vi "RG TAS v4c.vi"() -> ()   [LabVIEW 2017]
uses:
  Old Customer Code/Solar fuels TAS - DR/Sub VIs/global tas.vi
  <vilib>/Instr/_visa.llb/VISA Configure Serial Port (Instr).vi
  <vilib>/Analysis/NI_AALPro.lvlib
  <vilib>/Analysis/2dsp.llb/Decimate (single shot, DBL).vi
  <vilib>/Utility/file.llb/Write To Spreadsheet File (DBL).vi
  Optical Software Code Simplified/Modules/Monochromator/Oriel/Oriel (old drivers).lvlib
  Old Customer Code/Solar fuels TAS - DR/Sub VIs/Monochromator/global_Test.vi
  <vilib>/DAQmx/read.llb/DAQmx Read (Analog Wfm 1Chan NSamp).vi
  <vilib>/Analysis/NI_AALBase.lvlib
  <vilib>/Analysis/baseanly.llb/Mean (DBL).vi
  Old Customer Code/Solar fuels TAS - DR/Globals.vi
  <vilib>/Waveform/WDTOps.llb/WDT Index Channel DBL.vi
  <vilib>/Utility/file.llb/Write Delimited Spreadsheet (DBL).vi
panel:
  in  "Inspect Traces":bool
  out "DAQ Loop":i32
  out "Scope Error Counter":i32
  out "Scope time axis":dbl[](array[numeric])
  in  "Stop acquisition":bool
  out "Grating":i32
  in  "2b - Spectrum":bool
  in  "2a - Kinetic":bool
  in  "Stop":bool
  out "Btrace Readout Counter":i32=2
  in  "Stop Btrace Measurement":bool
  out "Readout Counter":i32=2
  in  "Stop Measurement":bool
  in  "Calculate Output Method":T1(ring)=enum."Reflectance"
  in  "Parameters":T2(tab)
  in  "Shutter flow control":u16(ring) items=["None"=0, "XON/XOFF"=1, "RTS/CTS"=2, "DTR/DSR"=4]
  in  "Shutter stop bits":u16(ring)=10 items=["1.0"=10, "1.5"=15, "2.0"=20]
  in  "Shutter parity":u16(ring) items=["None", "Odd", "Even", "Mark", "Space"]
  in  "Shutter data bits":u16=8 min=5 max=8 step=1
  in  "Shutter VISA resource name":refnum<visa-resource-name>="COM1"
  in  "Shutter baud rate":u32=9600
  in  "Shutter open string":string="+100 10\n"
  in  "1 - Move Shutter":bool
  in  "3 - Move mono":bool
  out "Current wavelength (Oriel)":dbl format="%#_13g"
  in  "Monochromator Type":bool=TRUE
  out "Start Wavelength":dbl min=0.0 format="%.3f"
  out "End Wavelength":dbl=100.0 min=0.0 format="%.3f"
  out "Interval Wavelength":dbl=10.0 min=0.0 format="%.3f"
  out "Current Wavelength (PTI)":dbl=300.0 min=300.0 max=2000.0 step=1.0
  in  "Is IR":bool caption="Grating"
  in  "Mono VISA name":refnum<visa-resource-name>
  in  "Mono 2 VISA name":refnum<visa-resource-name>
  out "DAQ dt":dbl=5e-06
  in  "DAQ End Time (s)":dbl=1.0
  in  "DAQ rate":i32=1250000
  in  "DAQ Trigger Level (V)":dbl=0.2
  out "DAQ Number of Samples":dbl=10000.0
  in  "DAQ average number of points":dbl=50.0
  out "DAQ final number of points":dbl
  in  "DAQ Input Channel":tag="Dev1/ai0"
  in  "100% Reflectance Standard (V)":dbl=1.0
  in  "DAQ Card":enum16{"USB-6211", "USB-6251"}(ring)=enum."USB-6251"
  in  "DAQ Input Config":i32(ring)=10106 items=["default"=-1, "RSE"=10083, "NRSE"=10078, "Differential"=10106, "Pseudodifferential"=12529]
  in  "Record Length":u32(ring)=10 items=["1000 points"=1, "10k points"=10, "100k points"=100, "1M points"=1000, "5M points"=5000, "10M points"=10000]
  in  "Acquisition Type":u16(ring)=2 items=["Sample", "Peak Detect", "Hi Res", "Envelope", "Average"]
  in  "Scope average\nnumber of points":dbl=1.0
  in  "Averages on scope":i32=1
  in  "Using TDS Scope?":bool
  in  "CH2 Impedance":u16(ring) items=["1M", "75", "50"]
  in  "CH1 Impedance":u16(ring)=2 items=["1M", "75", "50"]
  in  "Scope VISA resource name":refnum<visa-resource-name>="USB0::0x0699::0x0410::C022077::INSTR"
  in  "Scope Timeout (ms)":u32=30000
  in  "Channel TAS (0: Channel 1)":u16(ring) caption="Channel TAS" items=["Channel 1", "Channel 2", "Channel 3", "Channel 4", "Math", "Reference A", "Reference B", "Reference C", "Reference D"]
  in  "Channel TPC (0: Channel 1)":u16(ring)=1 caption="Channel TPC" items=["Channel 1", "Channel 2", "Channel 3", "Channel 4", "Math", "Reference A", "Reference B", "Reference C", "Reference D"]
  in  "Scope Timebase (per div)":dbl=0.0001 format="%^#_3e"
  in  "Trigger Source":u16(ring)=1 items=["Channel 1", "Channel 2", "Channel 3", "Channel 4", "AC Line", "Aux", "Digital Channel 0", "Digital Channel 1", "Digital Channel 2", "Digital Channel 3", "Digital Channel 4", "Digital Channel 5", "Digital Channel 6", "Digital Channel 7", "Digital Channel 8", "Digital Channel 9", "Digital Channel 10", "Digital Channel 11", "Digital Channel 12", "Digital Channel 13", "Digital Channel 14", "Digital Channel 15", "RF"]
  out "Final number of\nscope points":dbl=10000.0
  in  "Vertical Coupling TAS (1: DC)":u16(ring)=1 caption="Vertical Coupling TAS" items=["AC", "DC", "Ground"]
  in  "Probe Attenuation TAS (10.0)":dbl=1.0 caption="Probe Attenuation TAS"
  in  "Bandwidth CHTAS (0: FULL)":i32(ring) caption="Bandwidth CH TAS" items=["FULL", "250 MHz", "150 MHz", "20 MHz"]
  in  "Vertical Offset CH TAS (0.0 divs)":dbl caption="Vertical Offset CH TAS (in V)"
  in  "Vertical Range CH TAS (10.0 V)":dbl=0.5 caption="Vertical Range CH TAS"
  in  "Trigger Level (V)":dbl=0.25
  in  "Vertical Coupling TPC (1: DC)":u16(ring)=1 caption="Vertical Coupling TPC" items=["AC", "DC", "Ground"]
  in  "Probe Attenuation TPC (1.0)":dbl=1.0 caption="Probe Attenuation TPC"
  in  "Vertical Range TPC (10.0 V)":dbl=0.2 caption="Vertical Range TPC"
  in  "Bandwidth CH TPC (0: FULL)":i32(ring) caption="Bandwidth CH TPC" items=["FULL", "250 MHz", "150 MHz", "20 MHz"]
  in  "Vertical Offset CH TPC (0.0 divs)":dbl caption="Vertical Offset CH TPC (in V)"
  in  "TPC Multiplication factor":dbl=1.0
  out "Number of scope readouts":i32
  in  "Scope Channel Read":bool
  in  "LED on (s)":dbl
  in  "LED off (s)":dbl
  in  "PIA Mode":bool
  in  "LEDs (constant irrad.)":bool caption="LEDs"
  in  "DAQ LED line":string="Dev1/port1/line0"
  in  "Control LEDs?":bool
  out "Scope pretrigger points":dbl=1000.0
  out "Scope CH1 DOD data (A-B final)":waveform(dbl)(graph)
  out "Scope CH1 DOD data (A final)":waveform(dbl)(graph)={"t0"=timestamp(-4.0000000000040004e-05 s since 1904-01-01), "dt"=4.0000000000000003e-07, "Y"=array[10000 elements]}
  out "Scope CH2 data (final)":waveform(dbl)(graph)={"t0"=timestamp(-4.0000000000040004e-05 s since 1904-01-01), "dt"=4.0000000000000003e-07, "Y"=array[10000 elements]}
  out "DAQ DOD data (final)":waveform(dbl)(graph)={"t0"=timestamp(0 s since 1904-01-01), "dt"=5e-06, "Y"=array[10000 elements]}
  out "B trace (Channel1)":waveform(dbl)(graph)
  in  "Amplification Factor":dbl=400.0
  out "Background level (on Amp)":dbl=30.577247161746392
  out "Background level (V)":dbl=0.08993307988748939
  in  "Trace B ?":bool=TRUE
  out "Folder Created":bool
  in  "Sample Name":string="Sample"
  in  "TAS2014  Path":path=path "D:/Solar Fuels Data" caption="Folder"
  out "Path to Files":path=path "D:/Solar Fuels Data/Sample"
  out "Scope Average Channel2":waveform(dbl)(graph)={"t0"=timestamp(-4.0000000000040004e-05 s since 1904-01-01), "dt"=4.0000000000000003e-07, "Y"=array[10000 elements]}
  out "Scope Average Channel1":waveform(dbl)(graph)={"t0"=timestamp(-4.0000000000040004e-05 s since 1904-01-01), "dt"=4.0000000000000003e-07, "Y"=array[10000 elements]}
  out "DAQ Average Data":waveform(dbl)(graph)={"t0"=timestamp(0 s since 1904-01-01), "dt"=5e-06, "Y"=array[10000 elements]}
  in  "Number of Averages":i32=32
  out "DAQ Live Data":waveform(dbl)(graph)={"t0"=timestamp(0 s since 1904-01-01), "dt"=4.999999999999959e-06, "Y"=array[10000 elements]}
  # "Acquisition"
  # "Format: +100\\s20\\n OR \\F3\\002\\C1"
  # "Set COM ports for PTI\nmonochromators. If there\nis only 1 monochromator\npresent, leave Mono 2\nVISA name empty."
  # "DAQ Controls"
  # "DAQ Indicators"
  # "(Max = 250k/1.25M for\n6211/6251 DAQ cards)"
  # "Default is differential (connected ports are 15 and 16 on DAQ card).\n* For CH-TAS, input config should be RSE."
  # "Recommended Parameters for Different Scope Models"
  # "DPO3012"
  # "Record Length = 10k\nScope average number of points = 1"
  # "Acquisition Type = Hi Res\nAverages on scope = 1"
  # "DPO2012B"
  # "Record Length = 1M\nScope average number of points = 100"
  # "Acquisition Type = Average\nAverages on scope = 4"
  # "TDS3012C"
  # "Record Length = 10k\nScope average number of points = 1"
  # "Acquisition Type = Sample\nAverages on scope = 1"
  # "Channel 1"
  # "Channel 2"
  # "* For DPO2012B, impedance must be 1M for both channels!"
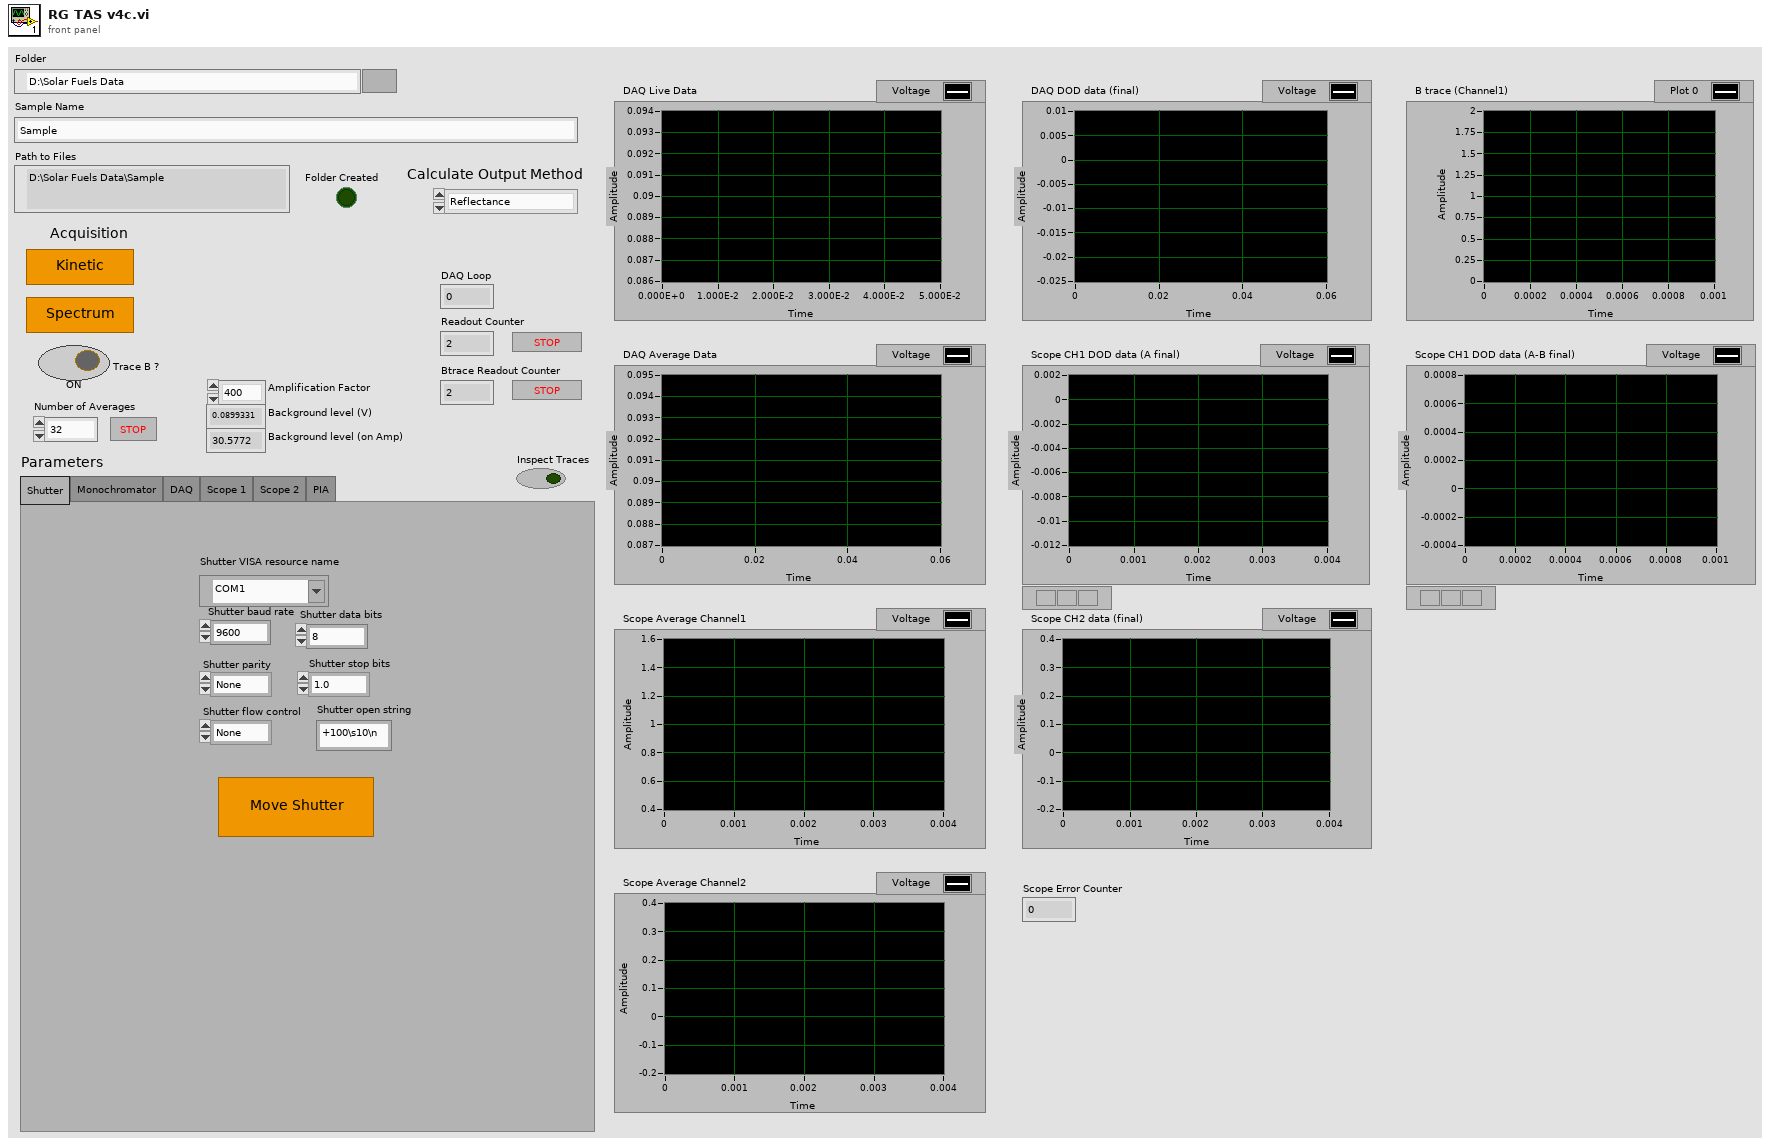
[diagram p1: front panel]
types:
  T1 = enum16{"Transmission", "Reflectance", "Kubelka-Munk"}
  T2 = enum32{"Shutter", "Monochromator", "DAQ", "Scope 1", "Scope 2", "PIA"}
  T3 = typedef "Monochromator Params.ctl" = cluster{"Type":enum32{"Oriel", "PTI"}, "Wavelength (nm)":dbl, "Wavelength (nm)":string, "Mono 2 VISA name":refnum<visa-resource-name>, "Mono VISA name":refnum<visa-resource-name>, "Start wavelength (nm)":dbl, "End wavelength (nm)":dbl, "Wavelength step (nm)":dbl}
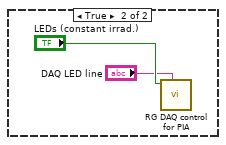
[diagram p2: hidden frame]
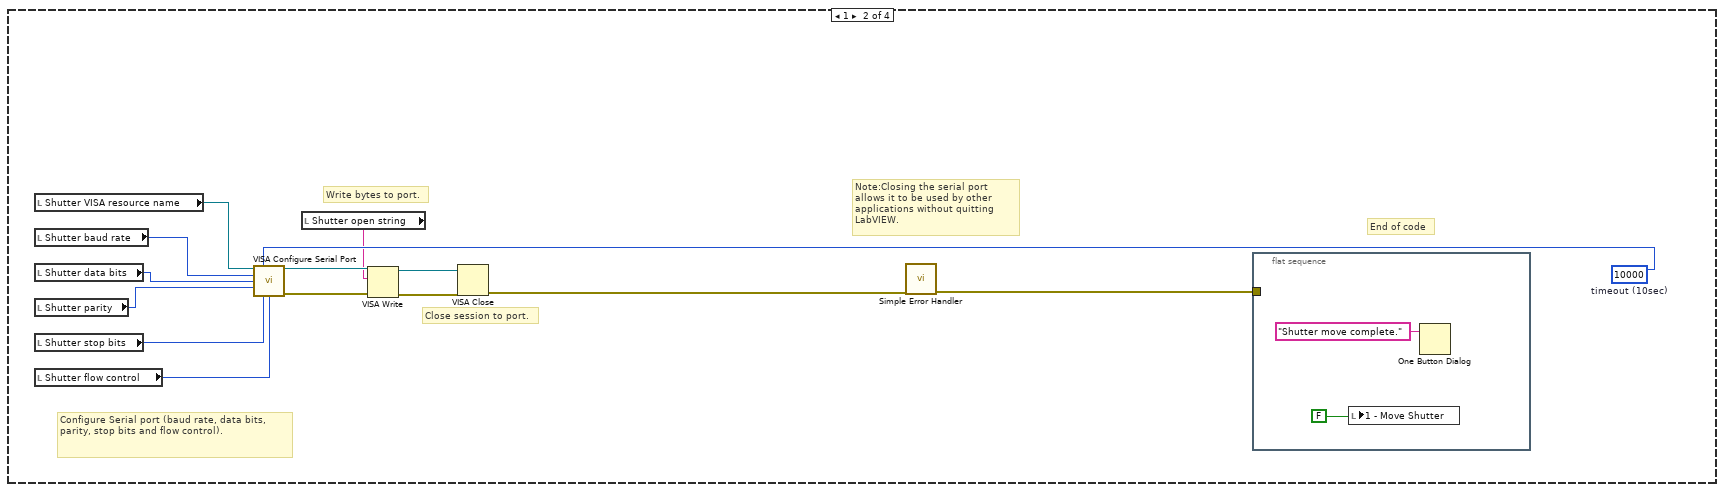
[diagram p4: hidden frame]
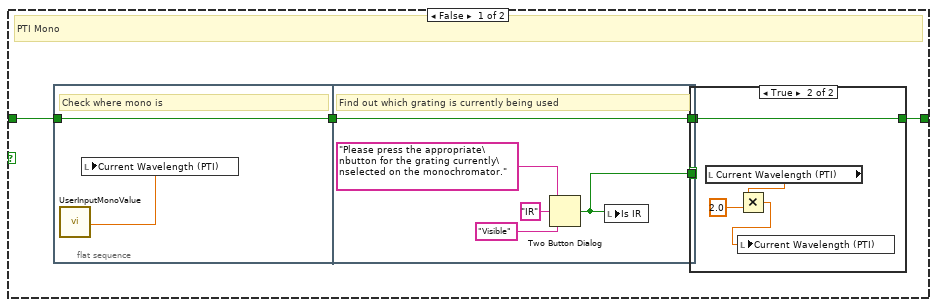
[diagram p5: hidden frame]
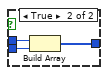
[diagram p8: hidden frame]
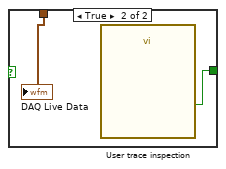
[diagram p9: hidden frame]
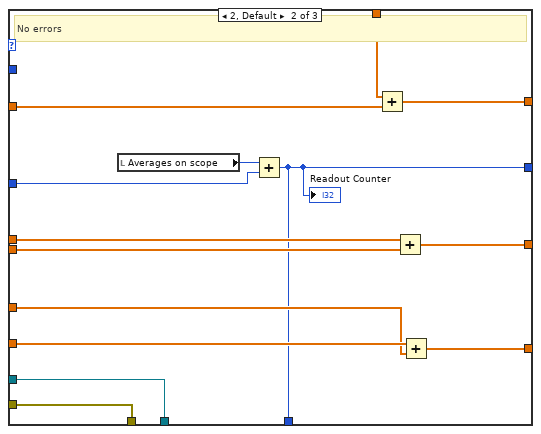
[diagram p11: hidden frame]
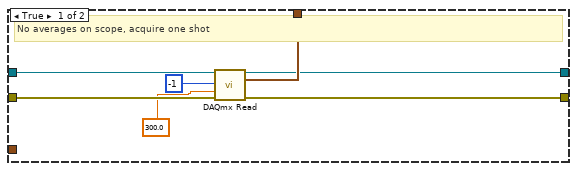
[diagram p13: hidden frame]
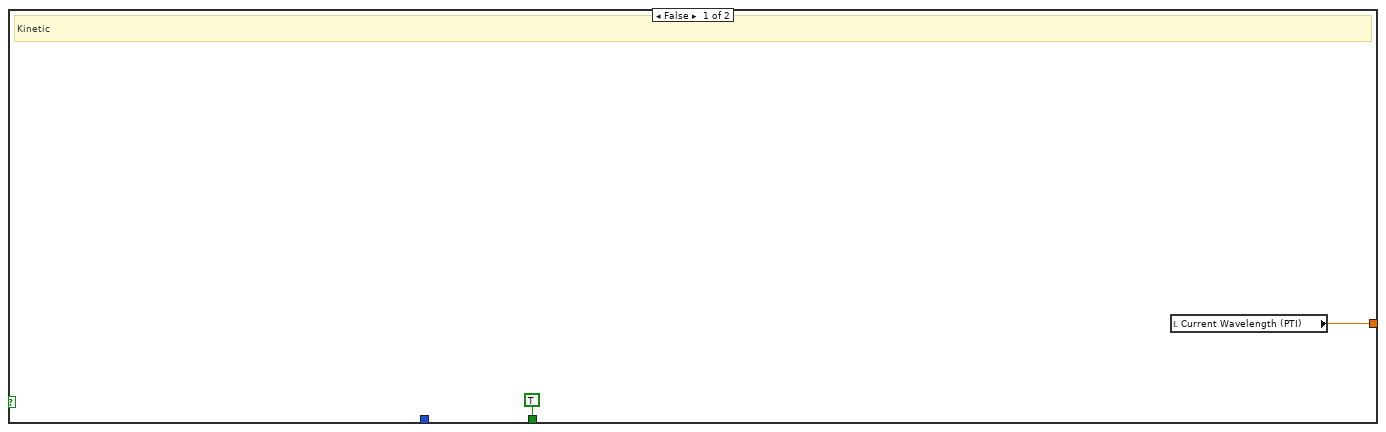
[diagram p14: hidden frame]
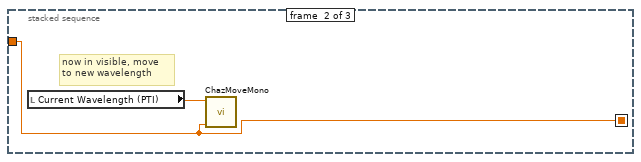
[diagram p16: hidden frame]
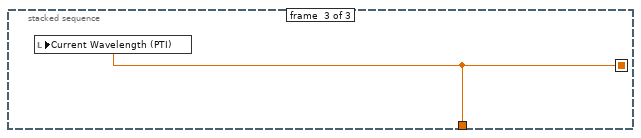
[diagram p17: hidden frame]
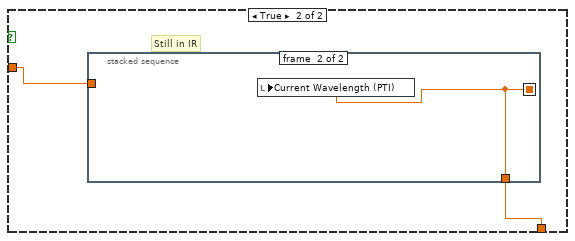
[diagram p18: hidden frame]
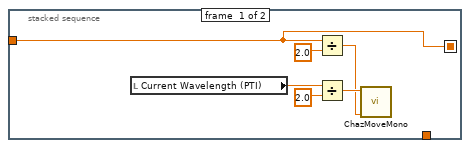
[diagram p19: hidden frame]
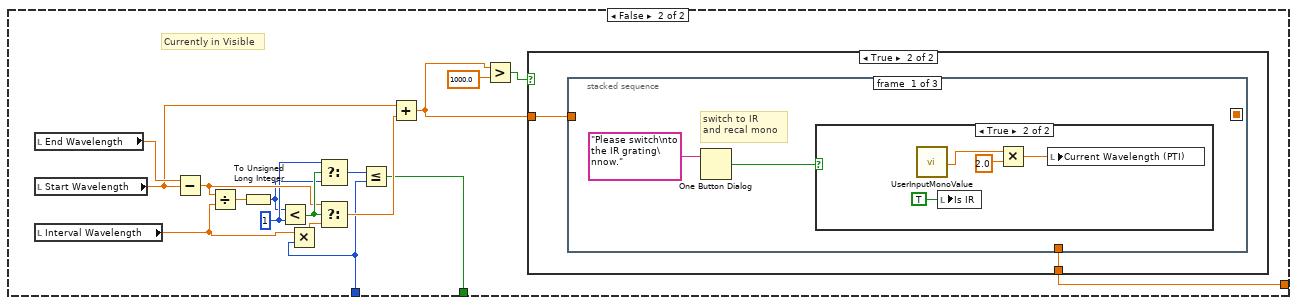
[diagram p20: hidden frame]
diagram:
  n1 = while {
    stop <- "Stop" stop-if-true
    # "True = Oriel"
    n2 = Or(x="2a - Kinetic", y="2b - Spectrum") -> (x .or. y?=w6:bool)
    n3 = Build Array(FALSE, "1 - Move Shutter", w6, "3 - Move mono") -> (w11:bool[])
    n4 = Search 1D Array(1D array=w11, element=TRUE) -> (index of element=w4:i32)  [unwired: 1 in]
    n5 = flat-sequence {
      tunnel: w4 -> [w37]
      tunnel: [w37] -> w3
      tunnel: "Monochromator Type" -> [w15]
      tunnel: [w15] -> w1
      frame #0 {
        # "Calculate DAQ parameters"
        # "Calculate Scope Parameters"
        n6 = case shown="False" "Control LEDs?" {
          frame False {
          }
          frame True {
            n7 = call "RG DAQ control for PIA.vi"("LED line"="DAQ LED line", "value"="LEDs (constant irrad.)") -> ()  [unwired: 9 in, 1 out]
          }
        }
        n8 = Multiply(x="DAQ End Time (s)", y=1.1) -> (x*y=w16:dbl)
        n9 = Multiply(x="Record Length", y=u32 1000) -> (x*y=w25:u32)
        n10 = Multiply(x="DAQ rate", y=w16) -> (x*y=w24:dbl)
        "DAQ Number of Samples" <- w24
        n11 = Reciprocal(x="DAQ rate") -> (1/x=→"DAQ dt":dbl)
        n12 = Divide(x="Number of Averages", y="Averages on scope") -> (x/y=→"Number of scope readouts":dbl)
        n13 = Divide(x=w25, y="Scope average\nnumber of points") -> (x/y=w29:dbl)
        "Final number of\nscope points" <- w29
        n14 = Divide(x=w29, y=10.0) -> (x/y=→"Scope pretrigger points":dbl)
        n15 = Wait (ms)(milliseconds to wait=u32 1000) -> ()  [unwired: 1 out]
        n16 = Divide(x=w24, y="DAQ average number of points") -> (x/y=→"DAQ final number of points":dbl)
        n17 = global write "global_Test.vi" "Mono VISA name"("Mono VISA name") -> ()
        n18 = global write "global_Test.vi" "Mono 2 VISA name"("Mono 2 VISA name") -> ()
      }
    }
    n19 = case shown="2" w3 {
      tunnel: w1 -> [_ _ w56 w1011]
      frame 0, Default {
      }
      frame 1 {
        w48 = u32 10000  # timeout (10sec)
        # "End of code"
        # "Note:Closing the serial port allows it to be used by other applications without quitting LabVIEW."
        # "Close session to port."
        # "Configure Serial port (baud rate, data bits, parity, stop bits and flow control)."
        # "Write bytes to port."
        n20 = local read "Shutter VISA resource name"() -> (w47:refnum<visa-resource-name>)
        n21 = local read "Shutter baud rate"() -> (w46:u32)
        n22 = local read "Shutter data bits"() -> (w45:u16)
        n23 = local read "Shutter parity"() -> (w44:u16)
        n24 = local read "Shutter stop bits"() -> (w43:u16)
        n25 = local read "Shutter flow control"() -> (w42:u16)
        n26 = call-poly "VISA Configure Serial Port"("VISA resource name"=w47, "timeout (10sec)"=w48, "baud rate (9600)"=w46, "data bits (8)"=w45, "parity (0:none)"=w44, "stop bits (10: 1 bit)"=w43, "flow control (0:none)"=w42) -> ("VISA resource name out"=w49:refnum<visa-resource-name>, "error out"=w50:errorcluster)  [unwired: 2 in, 5 out]
        n27 = local read "Shutter open string"() -> (w41:string)
        n28 = VISA Write(VISA resource name=w49, write buffer=w41, error in (no error)=w50) -> (VISA resource name out=w52:refnum<visa-resource-name>, error out=w53:errorcluster)  [unwired: 1 out]
        n29 = VISA Close(VISA resource name=w52, error in (no error)=w53) -> (error out=w51:errorcluster)
        n30 = call <vilib>:"Simple Error Handler.vi"("error in (no error)"=w51) -> ("error out"=w40:errorcluster)  [unwired: 1 in, 7 out]
        n31 = flat-sequence {
          tunnel: w40 -> [_]
          frame #0 {
            n32 = local write "1 - Move Shutter"(FALSE ("Move Shutter")) -> ()
            n33 = One Button Dialog(message="Shutter move complete.") -> ()  [unwired: 1 in, 1 out]
          }
        }
      }
      frame 2 {
        n34 = Build Path(base path="TAS2014  Path", name or relative path="Sample Name") -> (appended path=w67:path)
        n35 = call <vilib>:"Check if File or Folder Exists.vi"("path"=w67) -> ("file or folder exists?"=w66:bool, "dup path"=w65:path)  [unwired: 8 in, 1 out]
        n36 = case shown="True" w66 {
          tunnel: w65 -> [w1003 w1009]
          tunnel: [w1002 w1009] -> w60
          frame False {
            n37 = Create Folder(path (use dialog)=w1003) -> (created path=w1002:path)  [unwired: 2 in, 2 out]
            n38 = local write "Folder Created"(TRUE ("Folder Created")) -> ()
          }
          frame True {
            n39 = Two Button Dialog(message="Caution - folder already exists. Continue to overwrite data?", 1:"Yes, go for it!" ("F button name (\"Cancel\")"), 2:"No, help me!" ("T button name (\"OK\")")) -> (T button?=w1004:bool)
            n40 = local write "Folder Created"(FALSE ("Folder Created")) -> ()
            n41 = Stop(stop? (T)=w1004) -> ()
          }
        }
        "Path to Files" <- w60
        n42 = case shown="True" w56 {
          tunnel: w56 -> [w71 w86]
          tunnel: [w69 w85] -> w57
          frame False {
            # "PTI Mono"
            n43 = flat-sequence {
              tunnel: [w78] -> w72
              tunnel: w71 -> [w78]
              tunnel: w72 -> [w84]
              tunnel: [w84] -> w70
              tunnel: [w80] -> w68
              frame #0 {
                # "Check where mono is"
                n44 = call "UserInputMonoValue.vi"() -> ("Monochromator readout"=w79:dbl)  [unwired: 17 in, 2 out]
                n45 = local write "Current Wavelength (PTI)"(w79) -> ()
              }
              frame #1 {
                # "Find out which grating is currently being used"
                n46 = Two Button Dialog(message="Please press the appropriate\nbutton for the grating currently\nselected on the monochromator.", 1:"Visible" ("F button name (\"Cancel\")"), 2:"IR" ("T button name (\"OK\")")) -> (T button?=w80:bool)
                n47 = local write "Is IR"(w80) -> ()
              }
            }
            n48 = case shown="True" w68 {
              tunnel: w70 -> [w73 w77]
              tunnel: [w73 w77] -> w69
              frame False {
              }
              frame True {
                n49 = local read "Current Wavelength (PTI)"() -> (w75:dbl)
                n50 = Multiply(x=w75, y=2.0) -> (x*y=w74:dbl)
                n51 = local write "Current Wavelength (PTI)"(w74) -> ()
              }
            }
          }
          frame True {
            # "Oriel Mono"
            n52 = flat-sequence {
              tunnel: w86 -> [w90]
              tunnel: [w90] -> w85
              frame #0 {
                n53 = call "m_open.vi"() -> ("error out"=w91:errorcluster, "configuration file path copy"=w87:path)  [unwired: 2 in]
                n54 = call "GetWave.vi"("error in (no error)"=w91) -> ("error out"=w89:errorcluster, "Present Wavelength"=w88:dbl)  [unwired: 1 in]
                n55 = call "m_close.vi"("error in (no error)"=w89, "configuration file path"=w87) -> ()  [unwired: 2 out]
                n56 = local write "Current wavelength (Oriel)"(w88) -> ()
              }
            }
          }
        }
        n57 = local read "2b - Spectrum"() -> (w62:bool)
        n58 = global write "global tas.vi" "Root Path"(w60) -> ()
        n59 = case shown="True" w62 {
          tunnel: w60 -> [w95 w96]
          tunnel: [w95 w96] -> w58
          frame False {
          }
          frame True {
            n60 = call "RG Get Spectrum Wavelengths.vi"() -> ("Wavelength interval"=→"Interval Wavelength":i32, "End wavelength"=→"End Wavelength":i32, "Start wavelength"=→"Start Wavelength":i32)  [unwired: 9 in]
          }
        }
        n61 = flat-sequence {
          tunnel: [w92] -> w59
          tunnel: w58 -> [_]
          frame #0 {
            n62 = call "Prompt User for Input"() -> ("yes"=w92:bool)  [unwired: 18 in, 1 out]
          }
        }
        n63 = while {
          tunnel: [w207] -> w61
          tunnel: w59 -> [w202]
          tunnel: w57 -> [w195]
          i -> [w196]
          stop <- w225 stop-if-true
          w284 = TRUE  # Reset (True)
          w163 = 0
          w287 = FALSE  # ID Query (True)
          w320 = FALSE  # Enable Continuous Acquisition Mode (True)
          # "Some Maths to automatically output a stitched Scope-DAQ trace"
          # "Scope t0"
          # "Scope dt"
          # "DAQ index to make\nsure DAQ acquisition\nis finished before\ndoing B trace."
          # "Scope time\naxis"
          # "Scope time axis"
          # "Current wavelength"
          # "Current Wavelength"
          # "Make sure the 20s is waited before starting to acquire the data if shutter moves."
          # "Set time so that trigger\nis at t = 0"
          # "Get pre laser light level"
          # "Change cases for old TDS scope models because of differences in programming commands."
          # "Get pre laser light level (V) for DAQ and Scope"
          # "Disable time delay"
          # "Configure Timebase"
          # "Disable continous acquisition"
          # "Configure Trigger"
          # "If reading 2 channels, combine Channel A\n and Channel B so that both channels are read"
          # "Configure Channel B"
          # "Configure Channel A"
          # "Check the initial position of the shutter, and move if Doing Trace B and Spectrum"
          n64 = local read "2b - Spectrum"() -> (w199:bool)
          n65 = case shown="False" w195 {
            tunnel: [w561 w653] -> w224
            tunnel: [w558 w652] -> w222
            tunnel: [w560 w651] -> w206
            tunnel: w199 -> [w562 w650]
            tunnel: w196 -> [w563 w649]
            frame False {
              # "PTI Monochromator"
              n66 = flat-sequence {
                tunnel: w563 -> [w567]
                tunnel: w562 -> [w566]
                tunnel: [w565] -> w561
                tunnel: [w564] -> w559
                tunnel: [w648] -> w560
                tunnel: w559 -> [w648]
                tunnel: [w647] -> w558
                frame #0 {
                  n67 = case shown="True" w566 {
                    tunnel: w567 -> [_ w572]
                    tunnel: [TRUE w571] -> w565
                    tunnel: [w569 w570] -> w564
                    frame False {
                      # "Kinetic"
                      n68 = local read "Current Wavelength (PTI)"() -> (w569:dbl)
                    }
                    frame True {
                      # "Spectrum"
                      n69 = case shown="True" "Is IR" {
                        tunnel: w572 -> [w576 w612]
                        tunnel: [w577 w611] -> w571
                        tunnel: [w575 w610] -> w570
                        frame True {
                          w585 = u32 1 ("y")
                          # "Currently in IR"
                          n70 = local read "End Wavelength"() -> (w583:dbl)
                          n71 = local read "Start Wavelength"() -> (w581:dbl)
                          n72 = local read "Interval Wavelength"() -> (w578:dbl)
                          n73 = Subtract(x=w583, y=w581) -> (x-y=w586:dbl)
                          n74 = Divide(x=w586, y=w578) -> (x/y=w588:dbl)
                          n75 = To Unsigned Long Integer(number=w588) -> (unsigned 32bit integer=w584:u32)
                          n76 = Less?(x=w584, y=w585) -> (x < y?=w587:bool)
                          n77 = Multiply(x=w578, y=w576) -> (x*y=w579:dbl)
                          n78 = Select(t=w585, s=w587, f=w584) -> (s? t:f=w582:u32)
                          n79 = Select(t=w586, s=w587, f=w579) -> (s? t:f=w580:dbl)
                          n80 = Less Or Equal?(x=w582, y=w576) -> (x <= y?=w577:bool)
                          n81 = Add(x=w581, y=w580) -> (x+y=w574:dbl)
                          n82 = Greater?(x=w574, y=1000.0) -> (0:w589:bool)
                          n83 = case shown="False" w589 {
                            tunnel: [w592 w601] -> w575
                            tunnel: w574 -> [w591 w600]
                            frame False {
                              n84 = stacked-sequence {
                                seq-local: [_ w597 _] -> [_ _ w599]
                                tunnel: [_ _ w599] -> w592
                                tunnel: w591 -> [_ w597 _]
                                frame #0 {
                                # "switch to visible\nand recal mono"
                                n85 = One Button Dialog(message="Please switch\nto the visible grating\nnow.") -> (true=w593:bool)  [unwired: 1 in]
                                n86 = case shown="True" w593 {
                                frame False {
                                }
                                frame True {
                                n87 = call "UserInputMonoValue.vi"() -> ("Monochromator readout"=w595:dbl)  [unwired: 17 in, 2 out]
                                n88 = local write "Is IR"(FALSE ("Is IR")) -> ()
                                n89 = local write "Current Wavelength (PTI)"(w595) -> ()
                                }
                                }
                                }
                                frame #1 {
                                # "now in visible, move \nto new wavelength"
                                n90 = local read "Current Wavelength (PTI)"() -> (w598:dbl)
                                n91 = call "ChazMoveMono.vi"("Move to"=w597, "Current"=w598) -> ()  [unwired: 8 in, 2 out]
                                }
                                frame #2 {
                                n92 = local write "Current Wavelength (PTI)"(w599) -> ()
                                }
                              }
                            }
                            frame True {
                              # "Still in IR"
                              n93 = stacked-sequence {
                                seq-local: [w602 _] -> [_ w608]
                                tunnel: [_ w608] -> w601
                                tunnel: w600 -> [w602 _]
                                frame #0 {
                                n94 = local read "Current Wavelength (PTI)"() -> (w607:dbl)
                                n95 = Divide(x=w602, y=2.0) -> (x/y=w603:dbl)
                                n96 = Divide(x=w607, y=2.0) -> (x/y=w604:dbl)
                                n97 = call "ChazMoveMono.vi"("Move to"=w603, "Current"=w604) -> ()  [unwired: 8 in, 2 out]
                                }
                                frame #1 {
                                n98 = local write "Current Wavelength (PTI)"(w608) -> ()
                                }
                              }
                            }
                          }
                        }
                        frame False {
                          w620 = u32 1 ("y")
                          # "Currently in Visible"
                          n99 = local read "End Wavelength"() -> (w618:dbl)
                          n100 = local read "Start Wavelength"() -> (w616:dbl)
                          n101 = local read "Interval Wavelength"() -> (w613:dbl)
                          n102 = Subtract(x=w618, y=w616) -> (x-y=w621:dbl)
                          n103 = Divide(x=w621, y=w613) -> (x/y=w623:dbl)
                          n104 = To Unsigned Long Integer(number=w623) -> (unsigned 32bit integer=w619:u32)
                          n105 = Less?(x=w619, y=w620) -> (x < y?=w622:bool)
                          n106 = Multiply(x=w613, y=w612) -> (x*y=w614:dbl)
                          n107 = Select(t=w620, s=w622, f=w619) -> (s? t:f=w617:u32)
                          n108 = Select(t=w621, s=w622, f=w614) -> (s? t:f=w615:dbl)
                          n109 = Less Or Equal?(x=w617, y=w612) -> (x <= y?=w611:bool)
                          n110 = Add(x=w616, y=w615) -> (x+y=w609:dbl)
                          n111 = Greater?(x=w609, y=1000.0) -> (0:w624:bool)
                          n112 = case shown="True" w624 {
                            tunnel: [w627 w632] -> w610
                            tunnel: w609 -> [w626 w631]
                            frame False {
                              # "Still in Visible"
                              n113 = stacked-sequence {
                                seq-local: [w628 _] -> [_ w630]
                                tunnel: [_ w630] -> w627
                                tunnel: w626 -> [w628 _]
                                frame #0 {
                                n114 = local read "Current Wavelength (PTI)"() -> (w629:dbl)
                                n115 = call "ChazMoveMono.vi"("Move to"=w628, "Current"=w629) -> ()  [unwired: 8 in, 2 out]
                                }
                                frame #1 {
                                n116 = local write "Current Wavelength (PTI)"(w630) -> ()
                                }
                              }
                            }
                            frame True {
                              n117 = stacked-sequence {
                                seq-local: [_ w640 _] -> [_ _ w646]
                                tunnel: [_ _ w646] -> w632
                                tunnel: w631 -> [_ w640 _]
                                frame #0 {
                                # "switch to IR\nand recal mono"
                                n118 = One Button Dialog(message="Please switch\nto the IR grating\nnow.") -> (true=w633:bool)  [unwired: 1 in]
                                n119 = case shown="True" w633 {
                                frame False {
                                }
                                frame True {
                                n120 = call "UserInputMonoValue.vi"() -> ("Monochromator readout"=w637:dbl)  [unwired: 17 in, 2 out]
                                n121 = local write "Is IR"(TRUE ("Is IR")) -> ()
                                n122 = Multiply(x=w637, y=2.0) -> (x*y=w635:dbl)
                                n123 = local write "Current Wavelength (PTI)"(w635) -> ()
                                }
                                }
                                }
                                frame #1 {
                                # "now in IR, move \nto new wavelength"
                                n124 = local read "Current Wavelength (PTI)"() -> (w643:dbl)
                                n125 = Divide(x=w640, y=2.0) -> (x/y=w641:dbl)
                                n126 = Divide(x=w643, y=2.0) -> (x/y=w642:dbl)
                                n127 = global read "Globals.vi" "Monochromator"() -> (w639:T3)
                                n128 = call "ChazMoveMono.vi"("Monochromator"=w639, "Move to"=w641, "Current"=w642) -> ()  [unwired: 7 in, 2 out]
                                }
                                frame #2 {
                                n129 = local write "Current Wavelength (PTI)"(w646) -> ()
                                }
                              }
                            }
                          }
                        }
                      }
                    }
                  }
                }
                frame #1 {
                  n130 = call <vilib>:"General Error Handler.vi"() -> ("error out"=w647:errorcluster)  [unwired: 11 in, 4 out]
                }
              }
            }
            frame True {
              # "Oriel Monochromator"
              n131 = case shown="False" w650 {
                tunnel: [TRUE w683] -> w653
                tunnel: w649 -> [_ w670]
                tunnel: [w655 w668] -> w652
                tunnel: [w654 w667] -> w651
                frame False {
                  # "B trace OFF"
                  n132 = call "m_open.vi"() -> ("error out"=w657:errorcluster, "configuration file path copy"=w656:path)  [unwired: 2 in]
                  n133 = call "GetWave.vi"("error in (no error)"=w657) -> ("error out"=w665:errorcluster, "Present Wavelength"=w654:dbl)  [unwired: 1 in]
                  "Current wavelength (Oriel)" <- w654
                  n134 = Less Or Equal?(x=w654, y=590.0) -> (x <= y?=w664:bool)
                  n135 = Select(t=1.0, s=w664, f=2.0) -> (s? t:f=w661:dbl)
                  n136 = call "setgrat.vi"("error in (no error)"=w665, "Grating"=w661) -> ("error out"=w662:errorcluster)  [unwired: 1 in]
                  n137 = call "gowave.vi"("error in (no error)"=w662, "Destination Wavelength"=w654) -> ("error out"=w663:errorcluster)
                  n138 = call "m_close.vi"("error in (no error)"=w663, "configuration file path"=w656) -> ("error out"=w655:errorcluster)  [unwired: 1 out]
                }
                frame True {
                  w687 = u32 1 ("y")
                  # "B trace ON"
                  n139 = local read "End Wavelength"() -> (w685:dbl)
                  n140 = local read "Start Wavelength"() -> (w674:dbl)
                  n141 = local read "Interval Wavelength"() -> (w671:dbl)
                  n142 = Subtract(x=w685, y=w674) -> (x-y=w688:dbl)
                  n143 = Divide(x=w688, y=w671) -> (x/y=w690:dbl)
                  n144 = To Unsigned Long Integer(number=w690) -> (unsigned 32bit integer=w686:u32)
                  n145 = Less?(x=w686, y=w687) -> (x < y?=w689:bool)
                  n146 = Multiply(x=w671, y=w670) -> (x*y=w672:dbl)
                  n147 = Select(t=w687, s=w689, f=w686) -> (s? t:f=w684:u32)
                  n148 = Select(t=w688, s=w689, f=w672) -> (s? t:f=w673:dbl)
                  n149 = Less Or Equal?(x=w684, y=w670) -> (x <= y?=w683:bool)
                  n150 = Add(x=w674, y=w673) -> (x+y=w667:dbl)
                  n151 = call "m_open.vi"() -> ("error out"=w669:errorcluster, "configuration file path copy"=w682:path)  [unwired: 2 in]
                  n152 = Less Or Equal?(x=w667, y=590.0) -> (x <= y?=w675:bool)
                  n153 = local write "Current wavelength (Oriel)"(w667) -> ()
                  n154 = Select(t=1.0, s=w675, f=2.0) -> (s? t:f=w678:dbl)
                  n155 = call "setgrat.vi"("error in (no error)"=w669, "Grating"=w678) -> ("error out"=w677:errorcluster)  [unwired: 1 in]
                  n156 = call "gowave.vi"("error in (no error)"=w677, "Destination Wavelength"=w667) -> ("error out"=w676:errorcluster)
                  n157 = call "m_close.vi"("error in (no error)"=w676, "configuration file path"=w682) -> ("error out"=w668:errorcluster)  [unwired: 1 out]
                }
              }
            }
          }
          n158 = local read "Scope VISA resource name"() -> (w330:refnum<visa-resource-name>)
          n159 = local read "Trace B ?"() -> (w200:bool)
          n160 = And(x=w200, y=w199) -> (x .and. y?=w198:bool)
          n161 = Not Equal To 0?(x=w196) -> (x != 0?=w197:bool)
          n162 = And(x=w198, y=w197) -> (x .and. y?=w201:bool)
          n163 = Or(x=w202, y=w201) -> (x .or. y?=w203:bool)
          n164 = call "Initialize.vi"("error in (no error)"=w222, "Reset (True)"=w284, "ID Query (True)"=w287, "VISA resource name"=w330) -> ("error out"=w322:errorcluster, "VISA resource name out"=w321:refnum<visa-resource-name>)  [unwired: 6 in]
          n165 = local read "Scope Timeout (ms)"() -> (w157:u32)
          n166 = case shown="True" w203 {
            tunnel: [u32 0 ("millisecond timer value") w986] -> w142
            frame False {
            }
            frame True {
              w996 = u32 10000  # timeout (10sec)
              # "Note:Closing the serial port allows it to be used by other applications without quitting LabVIEW."
              # "Close session to port."
              # "Configure Serial port (baud rate, data bits, parity, stop bits and flow control)."
              # "Write bytes to port."
              n167 = call-poly "VISA Configure Serial Port"("VISA resource name"="Shutter VISA resource name", "timeout (10sec)"=w996, "baud rate (9600)"="Shutter baud rate", "data bits (8)"="Shutter data bits", "parity (0:none)"="Shutter parity", "stop bits (10: 1 bit)"="Shutter stop bits", "flow control (0:none)"="Shutter flow control") -> ("VISA resource name out"=w992:refnum<visa-resource-name>, "error out"=w991:errorcluster)  [unwired: 2 in, 5 out]
              n168 = VISA Write(VISA resource name=w992, write buffer="Shutter open string", error in (no error)=w991) -> (VISA resource name out=w989:refnum<visa-resource-name>, error out=w988:errorcluster)  [unwired: 1 out]
              n169 = VISA Close(VISA resource name=w989, error in (no error)=w988) -> (error out=w990:errorcluster)
              n170 = call <vilib>:"Simple Error Handler.vi"("error in (no error)"=w990) -> ()  [unwired: 1 in, 8 out]
              n171 = Wait (ms)(milliseconds to wait=u32 20000) -> (millisecond timer value=w986:u32)
            }
          }
          n172 = call "Configure Continuous Acquisition.vi"("error in (no error)"=w322, "Enable Continuous Acquisition Mode (T: Enable)"=w320, "VISA resource name"=w321) -> ("error out"=w161:errorcluster, "VISA resource name out"=w162:refnum<visa-resource-name>)  [unwired: 7 in]
          n173 = local read "Vertical Range CH TAS (10.0 V)"() -> (w315:dbl)
          n174 = local read "Vertical Offset CH TAS (0.0 divs)"() -> (w332:dbl)
          n175 = property class="Instr"(reference=w162, error in=w161, "General Settings:Timeout Value"=w157) -> (reference out=w160:refnum<visa-resource-name>, error out=w159:errorcluster)
          n176 = local read "Vertical Coupling TAS (1: DC)"() -> (w313:u16)
          n177 = local read "Bandwidth CHTAS (0: FULL)"() -> (w311:i32)
          n178 = local read "Probe Attenuation TAS (10.0)"() -> (w331:dbl)
          n179 = local read "Channel TAS (0: Channel 1)"() -> (w312:u16)
          n180 = Or(x=w224, y="Stop acquisition") -> (x .or. y?=w225:bool)
          n181 = local read "Vertical Offset CH TPC (0.0 divs)"() -> (w329:dbl)
          n182 = local read "Vertical Coupling TPC (1: DC)"() -> (w309:u16)
          n183 = local read "Probe Attenuation TPC (1.0)"() -> (w328:dbl)
          n184 = local read "Channel TPC (0: Channel 1)"() -> (w310:u16)
          n185 = local read "Vertical Range TPC (10.0 V)"() -> (w314:dbl)
          n186 = local read "Bandwidth CH TPC (0: FULL)"() -> (w308:i32)
          n187 = local read "Scope Timebase (per div)"() -> (w140:dbl)
          n188 = local read "Record Length"() -> (w305:u32)
          n189 = case shown="False" "Using TDS Scope?" {
            tunnel: w332 -> [w956 w984]
            tunnel: w331 -> [w955 w983]
            tunnel: w329 -> [w954 w982]
            tunnel: w328 -> [w953 w981]
            tunnel: w159 -> [w952 w980]
            tunnel: w160 -> [w951 w979]
            tunnel: w315 -> [w948 w976]
            tunnel: w314 -> [w947 w975]
            tunnel: w313 -> [w944 w972]
            tunnel: w312 -> [w943 w971]
            tunnel: w311 -> [w942 w970]
            tunnel: w310 -> [w941 w969]
            tunnel: w309 -> [w940 w968]
            tunnel: w308 -> [w939 w967]
            tunnel: w305 -> [w938 w966]
            tunnel: [w936 w964] -> w304
            tunnel: [w934 w962] -> w303
            tunnel: "CH1 Impedance" -> [w932 w960]
            tunnel: "CH2 Impedance" -> [w931 w959]
            tunnel: w140 -> [w930 w958]
            tunnel: 10.0 ("Position (10 %)") -> [w929 w957]
            frame True {
              n190 = call "RG Configure Channel TDS3012C.vi"("VISA resource name"=w951, "Input Impedance (0: 1M ohm)"=w932, "Channel (0: Channel 1)"=w943, "Vertical Coupling (1: DC)"=w944, "Probe Attenuation (1)"=w955, "error in (no error)"=w952, "Vertical Range (10.0 V)"=w948, "Vertical Offset (0.0 V)"=w956, "Bandwidth (0: FULL)"=w942) -> ("VISA resource name out"=w950:refnum<visa-resource-name>, "error out"=w949:errorcluster)  [unwired: 5 in]
              n191 = call "RG Configure Channel TDS3012C.vi"("VISA resource name"=w950, "Input Impedance (0: 1M ohm)"=w931, "Channel (0: Channel 1)"=w941, "Vertical Coupling (1: DC)"=w940, "Probe Attenuation (1)"=w953, "error in (no error)"=w949, "Vertical Range (10.0 V)"=w947, "Vertical Offset (0.0 V)"=w954, "Bandwidth (0: FULL)"=w939) -> ("VISA resource name out"=w945:refnum<visa-resource-name>, "error out"=w946:errorcluster)  [unwired: 5 in]
              n192 = call "RG Configure Timebase TDS3012C.vi"("Record Length (10: 10k points)"=w938, "error in (no error)"=w946, "Position (10 %)"=w929, "Timebase (0.0005 s)"=w930, "VISA resource name"=w945) -> ("error out"=w935:errorcluster, "VISA resource name out"=w937:refnum<visa-resource-name>)  [unwired: 5 in]
              n193 = call "RG Configure Delay TDS3012C.vi"("error in (no error)"=w935, "Enable Delay (T: Enable)"=FALSE, "VISA resource name"=w937) -> ("error out"=w934:errorcluster, "VISA resource name out"=w936:refnum<visa-resource-name>)  [unwired: 7 in]
            }
            frame False {
              n194 = call "Configure Channel.vi"("VISA resource name"=w979, "Input Impedance (0: 1M ohm)"=w960, "Channel (0: Channel 1)"=w971, "Vertical Coupling (1: DC)"=w972, "Probe Attenuation (1)"=w983, "error in (no error)"=w980, "Vertical Range (10.0 V)"=w976, "Vertical Offset (0.0 V)"=w984, "Bandwidth (0: FULL)"=w970) -> ("VISA resource name out"=w978:refnum<visa-resource-name>, "error out"=w977:errorcluster)  [unwired: 5 in]
              n195 = call "Configure Channel.vi"("VISA resource name"=w978, "Input Impedance (0: 1M ohm)"=w959, "Channel (0: Channel 1)"=w969, "Vertical Coupling (1: DC)"=w968, "Probe Attenuation (1)"=w981, "error in (no error)"=w977, "Vertical Range (10.0 V)"=w975, "Vertical Offset (0.0 V)"=w982, "Bandwidth (0: FULL)"=w967) -> ("VISA resource name out"=w973:refnum<visa-resource-name>, "error out"=w974:errorcluster)  [unwired: 5 in]
              n196 = call "Configure Timebase.vi"("Record Length (10: 10k points)"=w966, "error in (no error)"=w974, "Position (10 %)"=w957, "Timebase (0.0005 s)"=w958, "VISA resource name"=w973) -> ("error out"=w963:errorcluster, "VISA resource name out"=w965:refnum<visa-resource-name>)  [unwired: 5 in]
              n197 = call "Configure Delay.vi"("error in (no error)"=w963, "Enable Delay (T: Enable)"=FALSE, "VISA resource name"=w965) -> ("error out"=w962:errorcluster, "VISA resource name out"=w964:refnum<visa-resource-name>)  [unwired: 7 in]
            }
          }
          n198 = Multiply(x=w140, y=1800.0) -> (x*y=w138:dbl)
          n199 = flat-sequence {
            tunnel: [w340] -> w156
            tunnel: [w339] -> w155
            tunnel: [w338] -> w149
            tunnel: w142 -> [w337]
            tunnel: [w337] -> w141
            frame #0 {
              # "DAQ Setup acquisition"
              n200 = local read "DAQ Number of Samples"() -> (w341:dbl)
              n201 = local read "DAQ Trigger Level (V)"() -> (w348:dbl)
              n202 = local read "DAQ Input Channel"() -> (w349:tag)
              n203 = local read "DAQ rate"() -> (w342:i32)
              n204 = call "RG Configure DAQ auto Max input scale.vi"("input terminal configuration"="DAQ Input Config", "DAQ Card Type"="DAQ Card", "Sampling rate"=w342, "DAQ Trigger Level"=w348, "physical channel"=w349, "number of samples"=w341) -> ("error out"=w340:errorcluster, "task out"=w339:refnum<k21>)  [unwired: 4 in]
              n205 = Reciprocal(x=w342) -> (1/x=w343:dbl)
              n206 = Initialize Array(0.0 ("element"), w341) -> (w344:dbl[])
              n207 = Bundle By Name("Y"=w344, "dt"=w343) -> (w338:waveform(dbl))  [unwired: 1 in]
            }
          }
          n208 = Max & Min(x=w138, y=700.0) -> (max(x,y)=w136:dbl)  [unwired: 1 out]
          n209 = local read "Trigger Level (V)"() -> (w307:dbl)
          n210 = local read "Trigger Source"() -> (w306:u16)
          n211 = local read "DAQ final number of points"() -> (w168:dbl)
          n212 = case shown="False" "Scope Channel Read" {
            tunnel: [w350 w354] -> w323
            tunnel: w312 -> [w351 w353]
            tunnel: w310 -> [_ w352]
            frame False {
              n213 = Build Array(w351) -> (w350:u16[])
            }
            frame True {
              n214 = Build Array(w353, w352) -> (w354:u16[])
            }
          }
          n215 = local read "Averages on scope"() -> (w230:i32)
          n216 = call "RG Configure Trigger (Edge).vi"("VISA resource name"=w304, "Trigger Source (0: Channel 1)"=w306, "Trigger Level (0.0 V)"=w307, "error in (no error)"=w303) -> ("VISA resource name out"=w299:refnum<visa-resource-name>, "error out"=w300:errorcluster)  [unwired: 10 in]
          n217 = local read "Final number of\nscope points"() -> (w293:dbl)
          n218 = call "Configure Acquisition.vi"("error in (no error)"=w300, "Number of Waveform Acquisitions (16)"=w230, "Acquisition Type (0: Sample)"="Acquisition Type", "VISA resource name"=w299) -> ("error out"=w133:errorcluster, "VISA resource name out"=w135:refnum<visa-resource-name>)  [unwired: 6 in]
          n219 = local write "Scope Error Counter"(w163) -> ()
          n220 = flat-sequence {
            tunnel: w135 -> [w336]
            tunnel: [w336] -> w134
            tunnel: w133 -> [w335]
            tunnel: [w335] -> w132
            frame #0 {
              n221 = Wait (ms)(milliseconds to wait=u32 1000) -> ()  [unwired: 1 out]
            }
          }
          n222 = Initialize Array(0.0 ("element"), w168) -> (w166:dbl[])
          n223 = Initialize Array(0.0 ("element"), w293) -> (w165:dbl[])
          n224 = while {
            tunnel: w323 -> [w379]
            tunnel: [w378] -> w193
            shift-right: [w389] -> w174
            shift-left: w132 -> [w383]
            shift-right: [w385] -> w175
            shift-left: w134 -> [w384]
            shift-right: [w414] -> w290
            shift-left: w165 -> [w397]
            shift-right: [w415] -> w324
            shift-left: w166 -> [w395]
            shift-right: [w391] -> w151
            shift-left: w163 -> [w396]
            shift-right: [w393] -> w291
            shift-left: w165 -> [w392]
            tunnel: 0 -> [w390]
            tunnel: w156 -> [w374]
            tunnel: w155 -> [w375]
            tunnel: [w373] -> w154
            tunnel: [w372] -> w153
            tunnel: w149 -> [w371]
            tunnel: w141 -> [_]
            tunnel: w136 -> [w363]
            stop <- w398 stop-if-true
            w355 = TRUE ("element")
            n225 = flat-sequence {
              tunnel: w384 -> [w481]
              tunnel: [w478] -> w380
              tunnel: [w477] -> w381
              tunnel: [w485] -> w370
              tunnel: w383 -> [w480]
              tunnel: w375 -> [w476]
              tunnel: w374 -> [w475]
              tunnel: [w474] -> w373
              tunnel: [w473] -> w372
              tunnel: w371 -> [w472]
              tunnel: w363 -> [w459]
              frame #0 {
                # "To synch DAQ and scope acquisitions"
                n226 = local read "Averages on scope"() -> (w484:i32)
                n227 = local read "DAQ LED line"() -> (w463:string)
                n228 = Equal?(x=w484, y=1.0) -> (x = y?=w482:bool)
                n229 = call "Initiate.vi"("error in (no error)"=w480, "VISA resource name"=w481) -> ("error out"=w469:errorcluster, "VISA resource name out"=w471:refnum<visa-resource-name>)  [unwired: 8 in]
                n230 = Multiply(x="LED on (s)", y=1000.0) -> (x*y=w464:dbl)
                n231 = case shown="False" w482 {
                  tunnel: [w525 w531] -> w485
                  tunnel: w476 -> [w524 w530]
                  tunnel: w475 -> [w523 w529]
                  tunnel: [w521 w528] -> w474
                  tunnel: [w520 w527] -> w473
                  tunnel: w472 -> [_ w526]
                  frame True {
                    # "No averages on scope, acquire one shot"
                    n232 = call-poly <vilib>:"DAQmx Read.vi"("task/channels in"=w524, "number of samples per channel"=-1, "timeout"=300.0, "error in"=w523) -> ("task out"=w521:refnum<k21>, "data"=w525:waveform(dbl), "error out"=w520:errorcluster)  [unwired: 9 in]
                  }
                  frame False {
                    # "Averaging on scope, acquire multiple shots."
                    n233 = while {
                      shift-right: [w545] -> w531
                      shift-left: w526 -> [w544]
                      tunnel: w530 -> [w538]
                      tunnel: w529 -> [w537]
                      tunnel: [w534] -> w528
                      tunnel: [w533] -> w527
                      i -> [w541]
                      stop <- w543 stop-if-true
                      n234 = call-poly <vilib>:"DAQmx Read.vi"("task/channels in"=w538, "number of samples per channel"=-1, "timeout"=20.0, "error in"=w537) -> ("task out"=w534:refnum<k21>, "data"=w539:waveform(dbl), "error out"=w533:errorcluster)  [unwired: 9 in]
                      n235 = local read "Averages on scope"() -> (w542:i32)
                      n236 = Add(x=w541, y=1) -> (x+y=w535:i32)
                      "DAQ Loop" <- w535
                      n237 = Greater Or Equal?(x=w535, y=w542) -> (x >= y?=w543:bool)
                      n238 = Add(1:w544, 2:w539) -> (0:w545:waveform(dbl))  [unwired: 1 in, 1 out]
                    }
                  }
                }
                n239 = Multiply(x="LED off (s)", y=1000.0) -> (x*y=w460:dbl)
                n240 = case shown="True" "PIA Mode" {
                  tunnel: w471 -> [w487 w501]
                  tunnel: [w487 w495] -> w470
                  tunnel: w469 -> [w486 w500]
                  tunnel: [w486 w496] -> w468
                  tunnel: w464 -> [_ w499]
                  tunnel: w463 -> [_ w494]
                  tunnel: w460 -> [_ w493]
                  tunnel: w459 -> [_ w488]
                  frame False {
                  }
                  frame True {
                    n241 = flat-sequence {
                      tunnel: w494 -> [w510]
                      tunnel: w500 -> [w511]
                      tunnel: w501 -> [w512]
                      tunnel: [w512] -> w492
                      tunnel: [w511] -> w491
                      tunnel: [w510] -> w490
                      tunnel: [w509] -> w489
                      tunnel: w488 -> [w508]
                      tunnel: [w517] -> w498
                      tunnel: [w518] -> w497
                      tunnel: [w516] -> _
                      tunnel: w499 -> [w515]
                      tunnel: w492 -> [w517]
                      tunnel: w491 -> [w518]
                      tunnel: w490 -> [w513]
                      tunnel: w489 -> [_]
                      frame #0 {
                        n242 = Wait (ms)(milliseconds to wait=w508) -> (millisecond timer value=w509:u32)
                      }
                      frame #1 {
                        n243 = call "RG DAQ control for PIA.vi"("LED line"=w513, "value"=TRUE ("Initial value")) -> ()  [unwired: 9 in, 1 out]
                        n244 = Wait (ms)(milliseconds to wait=w515) -> (millisecond timer value=w516:u32)
                      }
                    }
                    n245 = flat-sequence {
                      tunnel: w498 -> [w507]
                      tunnel: [w507] -> w495
                      tunnel: [w506] -> _
                      tunnel: w493 -> [w505]
                      tunnel: w494 -> [w502]
                      tunnel: w497 -> [w503]
                      tunnel: [w503] -> w496
                      frame #0 {
                        n246 = call "RG DAQ control for PIA.vi"("LED line"=w502, "value"=FALSE ("Initial value")) -> ()  [unwired: 9 in, 1 out]
                        n247 = Wait (ms)(milliseconds to wait=w505) -> (millisecond timer value=w506:u32)
                      }
                    }
                  }
                }
                n248 = VISA Write(VISA resource name=w470, write buffer="*WAI", error in (no error)=w468) -> (VISA resource name out=w478:refnum<visa-resource-name>, error out=w477:errorcluster)  [unwired: 1 out]
              }
            }
            n249 = local read "Scope Timeout (ms)"() -> (w382:u32)
            n250 = local read "DAQ Number of Samples"() -> (w367:dbl)
            n251 = call "RG Fetch Waveforms from scope.vi"("error in (no error)"=w381, "Maximum Time (10000ms)"=w382, "Channels"=w379, "VISA resource name"=w380) -> ("error out"=w376:errorcluster, "Waveform Data"=w378:waveform(dbl)[], "VISA resource name out"=w377:refnum<visa-resource-name>)  [unwired: 5 in]
            n252 = Unbundle By Name(w376) -> ("status"=w388:bool)
            n253 = local read "Scope average\nnumber of points"() -> (w411:dbl)
            n254 = local read "DAQ rate"() -> (w364:i32)
            n255 = Multiply(x=w367, y=-0.1) -> (x*y=w365:dbl)
            n256 = local read "DAQ average number of points"() -> (w402:dbl)
            n257 = Divide(x=w365, y=w364) -> (x/y=w368:dbl)
            n258 = Split Signals(w378) -> (w409:dynamicdata, w408:dynamicdata)  [unwired: 2 in]
            n259 = To Time Stamp(1:w368) -> (0:w369:timestamp)
            n260 = Unbundle By Name(w370) -> ("Y"=w403:dbl[])
            n261 = call "Convert from Dynamic Data2"("Dynamic Data Type"=w409) -> ("Array"=w387:dbl[])  [unwired: 3 in]
            n262 = call "Convert from Dynamic Data3"("Dynamic Data Type"=w408) -> ("Array"=w407:dbl[])  [unwired: 3 in]
            n263 = Empty Array?(array=w387) -> (empty?=w386:bool)
            n264 = Bundle By Name(cluster=w370, "t0"=w369) -> (w356:waveform(dbl))
            n265 = case shown="False" "Inspect Traces" {
              tunnel: [TRUE w419] -> w357
              tunnel: w356 -> [w416 w418]
              frame False {
                n266 = local write "DAQ Live Data"(w416) -> ()
              }
              frame True {
                n267 = call "User trace inspection"() -> ("yes - keep it."=w419:bool)  [unwired: 18 in, 1 out]
                "DAQ Live Data" <- w418
              }
            }
            n268 = call-poly <vilib>:"Decimate (single shot).vi"("averaging"=TRUE, "decimating factor"=w402, "X"=w403) -> ("Decimated Array"=w394:dbl[])  [unwired: 7 in, 1 out]
            n269 = Not Or(1:w386, 2:w388) -> (0:w362:bool)
            n270 = call-poly <vilib>:"Decimate (single shot).vi"("averaging"=TRUE, "decimating factor"=w411, "X"=w387) -> ("Decimated Array"=w399:dbl[])  [unwired: 7 in, 1 out]
            n271 = call-poly <vilib>:"Decimate (single shot).vi"("averaging"=TRUE, "decimating factor"=w411, "X"=w407) -> ("Decimated Array"=w400:dbl[])  [unwired: 7 in, 1 out]
            n272 = Build Array(w355, w357, w355, w362) -> (w361:bool[])
            n273 = Search 1D Array(1D array=w361, element=FALSE) -> (index of element=w359:i32)  [unwired: 1 in]
            n274 = case shown="3" w359 {
              tunnel: [w425 w439 w451] -> w415
              tunnel: [w424 w438 w450] -> w414
              tunnel: [w422 w429 w445] -> w413
              tunnel: w400 -> [_ w437 _]
              tunnel: w399 -> [_ w436 _]
              tunnel: w397 -> [w424 w435 w450]
              tunnel: w396 -> [w422 w434 w445]
              tunnel: w395 -> [w425 w433 w451]
              tunnel: w394 -> [_ w432 _]
              tunnel: [w423 w431 w449] -> w393
              tunnel: w392 -> [w423 w430 w449]
              tunnel: [w422 w429 w445] -> w391
              tunnel: w390 -> [_ _ w447]
              tunnel: w376 -> [w420 w428 w443]
              tunnel: [w420 w428 w441] -> w389
              tunnel: w377 -> [w421 w427 w444]
              tunnel: [w421 w427 w440] -> w385
              frame 1 {
                # "User Rejects Trace"
              }
              frame 2, Default {
                # "No errors"
                n275 = local read "Averages on scope"() -> (w426:i32)
                n276 = Add(x=w426, y=w434) -> (x+y=w429:i32)
                "Readout Counter" <- w429
                n277 = Add(x=w432, y=w433) -> (x+y=w439:dbl[])
                n278 = Add(x=w435, y=w436) -> (x+y=w438:dbl[])
                n279 = Add(x=w437, y=w430) -> (x+y=w431:dbl[])
              }
              frame 3 {
                # "Scope Error Detected"
                n280 = flat-sequence {
                  tunnel: w444 -> [w452]
                  tunnel: w443 -> [w453]
                  tunnel: [w452] -> w442
                  tunnel: w442 -> [w458]
                  tunnel: [w455] -> w441
                  tunnel: [w454] -> w440
                  frame #0 {
                    n281 = call "Close.vi"("error in (no error)"=w453, "VISA resource name"=w452) -> ()  [unwired: 9 in, 1 out]
                  }
                  frame #1 {
                    w457 = FALSE ("ID Query (True)")
                    n282 = call "Initialize.vi"("error in (no error)"=errorcluster {"status"=FALSE, "code"=0, "source"=""}, "Reset (True)"=w457, "ID Query (True)"=w457, "VISA resource name"=w458) -> ("error out"=w455:errorcluster, "VISA resource name out"=w454:refnum<visa-resource-name>)  [unwired: 6 in]
                  }
                }
                n283 = Add(x=w447, y=1.0) -> (x+y=→"Scope Error Counter":dbl)
              }
            }
            n284 = local read "Number of Averages"() -> (w406:i32)
            n285 = Greater Or Equal?(x=w413, y=w406) -> (x >= y?=w405:bool)
            n286 = Or(x=w405, y="Stop Measurement") -> (x .or. y?=w398:bool)
          }
          n287 = call-poly <vilib>:"Index Waveform Array.vi"("index"=0, "waveform array"=w193) -> ("waveform"=w191:waveform(dbl))  [unwired: 8 in, 1 out]
          n288 = Unbundle By Name(w191) -> ("t0"=w173:timestamp, "dt"=w172:dbl)
          n289 = local read "Record Length"() -> (w187:u32)
          n290 = To Double Precision Float(number=w173) -> (double precision float=w190:dbl)
          n291 = Multiply(x=w187, y=1000.0) -> (x*y=w189:dbl)
          n292 = local read "Scope average\nnumber of points"() -> (w184:dbl)
          n293 = for {
            N: w189 -> [_]
            tunnel: w190 -> [w557]
            tunnel: w172 -> [w555]
            tunnel: [w553] -> w186 mode=indexing
            i -> [w556]
            n294 = Multiply(x=w555, y=w556) -> (x*y=w554:dbl)
            n295 = Add(x=w557, y=w554) -> (x+y=w553:dbl)
          }
          n296 = call-poly <vilib>:"Decimate (single shot).vi"("averaging"=TRUE, "decimating factor"=w184, "X"=w186) -> ("Decimated Array"=w104:dbl[])  [unwired: 7 in, 1 out]
          "Scope time axis" <- w104
          n297 = call <vilib>:"DAQmx Clear Task.vi"("task in"=w154, "error in"=w153) -> ()  [unwired: 13 in, 1 out]
          n298 = local read "Averages on scope"() -> (w152:i32)
          n299 = Divide(x=w151, y=w152) -> (x/y=w150:dbl)
          n300 = Divide(x=w291, y=w150) -> (x/y=w333:dbl[])
          n301 = Divide(x=w290, y=w150) -> (x/y=w226:dbl[])
          n302 = local read "DAQ final number of points"() -> (w148:dbl)
          n303 = Bundle By Name("Y"=w333, "t0"=w173, "dt"=w172) -> (→"Scope Average Channel2":waveform(dbl))  [unwired: 1 in]
          n304 = Bundle By Name("Y"=w226, "t0"=w173, "dt"=w172) -> (→"Scope Average Channel1":waveform(dbl))  [unwired: 1 in]
          n305 = local read "DAQ average number of points"() -> (w294:dbl)
          n306 = Divide(x=w324, y=w151) -> (x/y=w194:dbl[])
          n307 = local read "DAQ dt"() -> (w295:dbl)
          n308 = Multiply(x=w148, y=-0.1) -> (x*y=w145:dbl)
          n309 = Multiply(x=w295, y=w294) -> (x*y=w146:dbl)
          n310 = Multiply(x=w145, y=w146) -> (x*y=w143:dbl)
          n311 = To Time Stamp(1:w143) -> (0:w144:timestamp)
          n312 = local read "DAQ final number of points"() -> (w302:dbl)
          n313 = Bundle By Name("Y"=w194, "t0"=w144, "dt"=w146) -> (→"DAQ Average Data":waveform(dbl))  [unwired: 1 in]
          n314 = Multiply(x=w302, y=0.075) -> (x*y=w297:dbl)
          n315 = Round To Nearest(number=w297) -> (nearest integer value=w296:dbl)
          n316 = Array Subset(array=w194, index=0, length=w296) -> (w318:dbl[])
          n317 = local read "Amplification Factor"() -> (w316:dbl)
          n318 = Add Array Elements(numeric array=w318) -> (sum=w317:dbl)
          n319 = Divide(x=w317, y=w296) -> (x/y=w170:dbl)
          n320 = Multiply(x=w170, y=w316) -> (x*y=w171:dbl)
          n321 = local write "Background level (on Amp)"(w171) -> ()
          n322 = local write "Background level (V)"(w170) -> ()
          n323 = local read "DAQ Number of Samples"() -> (w177:dbl)
          n324 = for {
            N: w177 -> [_]
            tunnel: [w547] -> w178 mode=indexing
            i -> [w552]
            n325 = local read "DAQ Number of Samples"() -> (w551:dbl)
            n326 = Divide(x=w551, y=10.0) -> (x/y=w549:dbl)
            n327 = local read "DAQ dt"() -> (w546:dbl)
            n328 = Subtract(x=w552, y=w549) -> (x-y=w548:dbl)
            n329 = Multiply(x=w548, y=w546) -> (x*y=w547:dbl)
          }
          n330 = local read "DAQ average number of points"() -> (w180:dbl)
          n331 = Number To Decimal String(number=w206, width (-)=i16 3) -> (decimal integer string=w205:string)
          n332 = call-poly <vilib>:"Decimate (single shot).vi"("averaging"=TRUE, "decimating factor"=w180, "X"=w178) -> ("Decimated Array"=w176:dbl[])  [unwired: 7 in, 1 out]
          n333 = Concatenate Strings(w205, "nm Scope CH2 (raw data).txt") -> (w218:string)
          n334 = global read "global tas.vi" "Root Path"() -> (w282:path)
          n335 = Build Array(w176, w194) -> (w283:dbl[][])
          n336 = Build Array(w104, w226) -> (w273:dbl[][])
          n337 = global read "global tas.vi" "Root Path"() -> (w277:path)
          n338 = Concatenate Strings(w205, "nm DAQ (raw data).txt") -> (w221:string)
          n339 = global read "global tas.vi" "Root Path"() -> (w204:path)
          n340 = Build Array(w104, w333) -> (w278:dbl[][])
          n341 = Concatenate Strings(w205, "nm Scope CH1 (raw data).txt") -> (w216:string)
          n342 = Build Path(base path=w282, name or relative path=w221) -> (appended path=w281:path)
          n343 = Build Path(base path=w277, name or relative path=w218) -> (appended path=w276:path)
          n344 = Build Path(base path=w204, name or relative path=w216) -> (appended path=w272:path)
          n345 = call-poly <vilib>:"Write To Spreadsheet File.vi"("transpose? (no:F)"=TRUE, "format (%.3f)"="%.9f", "2D data"=w283, "file path (dialog if empty)"=w281) -> ()  [unwired: 4 in, 1 out]
          n346 = call-poly <vilib>:"Write To Spreadsheet File.vi"("transpose? (no:F)"=TRUE, "format (%.3f)"="%.9f", "2D data"=w273, "file path (dialog if empty)"=w272) -> ()  [unwired: 4 in, 1 out]
          n347 = call-poly <vilib>:"Write To Spreadsheet File.vi"("transpose? (no:F)"=TRUE, "format (%.3f)"="%.9f", "2D data"=w278, "file path (dialog if empty)"=w276) -> ()  [unwired: 4 in, 1 out]
          n348 = flat-sequence {
            tunnel: w205 -> [w692]
            tunnel: w204 -> [w691]
            tunnel: w169 -> [_]
            frame #0 {
              # "Write parameters file after values have been calculated."
              n349 = Build Array("Number of Averages", "Scope acq. type", "Number of averages on scope", "Scope average number of points", "Scope timebase (s)", "Scope CH1 vertical scale per div (V)", "Scope CH2 vertical scale per div (V)", "Background level on amp (V)", "DAQ sampling rate (Hz)", "DAQ average number of points", "Background level on DAQ (V)", "Amplification factor", "100% Reflection Reference Signal (V)" ("element"), "Output calculation Method" ("element")) -> (w716:string[])
              n350 = Concatenate Strings(w692, "nm Parameters.txt") -> (w694:string)
              n351 = local read "Scope Timebase (per div)"() -> (w708:dbl)
              n352 = local read "Averages on scope"() -> (w707:i32)
              n353 = local read "DAQ rate"() -> (w712:i32)
              n354 = local read "Acquisition Type"() -> (w725:u16)
              n355 = Build Path(base path=w691, name or relative path=w694) -> (appended path=w718:path)
              n356 = local read "Scope average\nnumber of points"() -> (w706:dbl)
              n357 = local read "Vertical Range CH TAS (10.0 V)"() -> (w709:dbl)
              n358 = local read "Vertical Range TPC (10.0 V)"() -> (w710:dbl)
              n359 = local read "Background level (on Amp)"() -> (w711:dbl)
              n360 = local read "DAQ average number of points"() -> (w713:dbl)
              n361 = local read "Background level (V)"() -> (w714:dbl)
              n362 = local read "Amplification Factor"() -> (w715:dbl)
              n363 = local read "100% Reflectance Standard (V)"() -> (w727:dbl)
              n364 = local read "Calculate Output Method"() -> (w729:T1)
              n365 = local read "Readout Counter"() -> (w723:i32)
              n366 = Build Array(w723, w725, w707, w706, w708, w709, w710, w711, w712, w713, w714, w715, w727, w729) -> (w717:dbl[])
              n367 = Number To Fractional String(number=w717) -> (F-format string=w693:string[])  [unwired: 3 in]
              n368 = Build Array(w716, w693) -> (w719:string[][])
              n369 = Array To Spreadsheet String(array=w719, 3:"%s" ("format string")) -> (spreadsheet string=w721:string)  [unwired: 1 in]
              n370 = Write to Text File(file (use dialog)=w718, text=w721) -> ()  [unwired: 2 in, 3 out]
            }
          }
          n371 = local read "Calculate Output Method"() -> (w238:T1)
          n372 = local read "TPC Multiplication factor"() -> (w258:dbl)
          n373 = case shown="\"Kubelka-Munk\"" w238 {
            tunnel: w194 -> [w760 w765 w783]
            tunnel: [w759 w763 w775] -> w109
            tunnel: w170 -> [w758 w762 w766]
            frame "Transmission" {
              # "Background level on DAQ"
              # "Calculate output as: deltaOD = log(T/T')"
              n374 = Divide(x=w758, y=w760) -> (x/y=w761:dbl[])
              n375 = Logarithm Base 10(1:w761) -> (0:w759:dbl[])
            }
            frame "Reflectance" {
              # "Calculate output as: Transient abs. = 1 - RT = (Rbkg - R(t)) / Rbkg"
              n376 = Subtract(x=w762, y=w765) -> (x-y=w764:dbl[])
              n377 = Divide(x=w764, y=w762) -> (x/y=w763:dbl[])
            }
            frame "Kubelka-Munk" {
              # "Calculate output from\nKM = (1-Rrelative)^2/(2*Rrelative)"
              n378 = local read "100% Reflectance Standard (V)"() -> (w782:dbl)
              n379 = Divide(x=w783, y=w782) -> (x/y=w768:dbl[])
              n380 = Subtract(x=1.0, y=w768) -> (x-y=w770:dbl[])
              n381 = Divide(x=w766, y=w782) -> (x/y=w777:dbl)
              n382 = Square(x=w770) -> (x^2=w771:dbl[])
              n383 = Subtract(x=1.0, y=w777) -> (x-y=w780:dbl)
              n384 = Multiply(x=w768, y=2.0) -> (x*y=w772:dbl[])
              n385 = Square(x=w780) -> (x^2=w779:dbl)
              n386 = Divide(x=w771, y=w772) -> (x/y=w767:dbl[])
              n387 = Multiply(x=w777, y=2.0) -> (x*y=w778:dbl)
              n388 = Divide(x=w779, y=w778) -> (x/y=w774:dbl)
              n389 = Subtract(x=w767, y=w774) -> (x-y=w775:dbl[])
            }
          }
          n390 = local read "DAQ average number of points"() -> (w231:dbl)
          n391 = local read "DAQ final number of points"() -> (w242:dbl)
          n392 = Multiply(x=w333, y=w258) -> (x*y=w125:dbl[])
          n393 = local read "DAQ dt"() -> (w232:dbl)
          n394 = local read "Scope pretrigger points"() -> (w246:dbl)
          n395 = Multiply(x=w232, y=w231) -> (x*y=w233:dbl)
          n396 = Divide(x=w242, y=-10.0) -> (x/y=w241:dbl)
          n397 = Multiply(x=w241, y=w233) -> (x*y=w240:dbl)
          n398 = To Time Stamp(1:w240) -> (0:w239:timestamp)
          n399 = Multiply(x=w246, y=0.75) -> (x*y=w245:dbl)
          n400 = Bundle By Name("Y"=w125, "t0"=w173, "dt"=w172) -> (→"Scope CH2 data (final)":waveform(dbl))  [unwired: 1 in]
          n401 = Array Subset(array=w226, index=0, length=w245) -> (w249:dbl[])
          n402 = Add Array Elements(numeric array=w249) -> (sum=w250:dbl)
          n403 = Divide(x=w250, y=w245) -> (x/y=w251:dbl)
          n404 = Subtract(x=w226, y=w251) -> (x-y=w237:dbl[])
          n405 = local read "Calculate Output Method"() -> (w234:T1)
          n406 = Bundle By Name("Y"=w109, "t0"=w239, "dt"=w233) -> (→"DAQ DOD data (final)":waveform(dbl))  [unwired: 1 in]
          n407 = Add(x=w237, y=w171) -> (x+y=w236:dbl[])
          n408 = case shown="\"Kubelka-Munk\"" w234 {
            tunnel: w236 -> [w731 w737 w756]
            tunnel: [w730 w734 w749] -> w235
            frame "Transmission" {
              # "Calculate output as: deltaOD = log(T/T')"
              n409 = local read "Background level (on Amp)"() -> (w732:dbl)
              n410 = Divide(x=w732, y=w731) -> (x/y=w733:dbl[])
              n411 = Logarithm Base 10(1:w733) -> (0:w730:dbl[])
            }
            frame "Reflectance" {
              # "Calculate output as: Transient abs. = 1 - RT = (Rbkg - R(t)) / Rbkg"
              n412 = local read "Background level (on Amp)"() -> (w736:dbl)
              n413 = Subtract(x=w736, y=w737) -> (x-y=w735:dbl[])
              n414 = Divide(x=w735, y=w736) -> (x/y=w734:dbl[])
            }
            frame "Kubelka-Munk" {
              # "Calculate output from\nKM = (1-Rrelative)^2/(2*Rrelative)"
              n415 = local read "100% Reflectance Standard (V)"() -> (w739:dbl)
              n416 = local read "Amplification Factor"() -> (w740:dbl)
              n417 = local read "Background level (on Amp)"() -> (w757:dbl)
              n418 = Multiply(x=w739, y=w740) -> (x*y=w738:dbl)
              n419 = Divide(x=w756, y=w738) -> (x/y=w742:dbl[])
              n420 = Subtract(x=1.0, y=w742) -> (x-y=w744:dbl[])
              n421 = Divide(x=w757, y=w738) -> (x/y=w751:dbl)
              n422 = Square(x=w744) -> (x^2=w745:dbl[])
              n423 = Subtract(x=1.0, y=w751) -> (x-y=w754:dbl)
              n424 = Multiply(x=w742, y=2.0) -> (x*y=w746:dbl[])
              n425 = Square(x=w754) -> (x^2=w753:dbl)
              n426 = Divide(x=w745, y=w746) -> (x/y=w741:dbl[])
              n427 = Multiply(x=w751, y=2.0) -> (x*y=w752:dbl)
              n428 = Divide(x=w753, y=w752) -> (x/y=w748:dbl)
              n429 = Subtract(x=w741, y=w748) -> (x-y=w749:dbl[])
            }
          }
          n430 = local read "DAQ Number of Samples"() -> (w247:dbl)
          n431 = for {
            N: w247 -> [_]
            tunnel: [w785] -> w183 mode=indexing
            i -> [w790]
            n432 = local read "DAQ Number of Samples"() -> (w789:dbl)
            n433 = Divide(x=w789, y=10.0) -> (x/y=w787:dbl)
            n434 = local read "DAQ dt"() -> (w784:dbl)
            n435 = Subtract(x=w790, y=w787) -> (x-y=w786:dbl)
            n436 = Multiply(x=w786, y=w784) -> (x*y=w785:dbl)
          }
          n437 = Number To Decimal String(number=w206, width (-)=i16 3) -> (decimal integer string=w128:string)
          n438 = local read "DAQ average number of points"() -> (w181:dbl)
          n439 = Concatenate Strings(w128, "nm Scope CH1 (final A).txt") -> (w209:string)
          n440 = Build Array(w104, w125) -> (w264:dbl[][])
          n441 = global read "global tas.vi" "Root Path"() -> (w255:path)
          n442 = Concatenate Strings(w128, "nm Scope CH2 (final).txt") -> (w211:string)
          n443 = global read "global tas.vi" "Root Path"() -> (w263:path)
          n444 = Build Path(base path=w255, name or relative path=w209) -> (appended path=w254:path)
          n445 = Array Size(array=w104) -> (size(s)=w123:i32)
          n446 = Build Path(base path=w263, name or relative path=w211) -> (appended path=w262:path)
          n447 = call-poly <vilib>:"Decimate (single shot).vi"("averaging"=TRUE, "decimating factor"=w181, "X"=w183) -> ("Decimated Array"=w107:dbl[])  [unwired: 7 in, 1 out]
          n448 = Multiply(x=w123, y=0.95) -> (x*y=w122:dbl)
          n449 = call-poly <vilib>:"Write To Spreadsheet File.vi"("transpose? (no:F)"=TRUE, "format (%.3f)"="%.9f", "2D data"=w264, "file path (dialog if empty)"=w262) -> ()  [unwired: 4 in, 1 out]
          n450 = Bundle By Name("Y"=w235, "t0"=w173, "dt"=w172) -> (w228:waveform(dbl))  [unwired: 1 in]
          "Scope CH1 DOD data (A final)" <- w228
          n451 = Build Array(w107, w109) -> (w257:dbl[][])
          n452 = global read "global tas.vi" "Root Path"() -> (w266:path)
          n453 = Build Array(w104, w235) -> (w256:dbl[][])
          n454 = Array Subset(array=w104, index=w122) -> (w120:dbl[])  [unwired: 1 in]
          n455 = Array Max & Min(array=w120) -> (max value=w119:dbl, min value=w118:dbl)  [unwired: 2 out]
          n456 = call-poly <vilib>:"Write To Spreadsheet File.vi"("transpose? (no:F)"=TRUE, "format (%.3f)"="%.9f", "2D data"=w256, "file path (dialog if empty)"=w254) -> ("new file path (Not A Path if cancelled)"=w169:path)  [unwired: 4 in]
          n457 = Concatenate Strings(w128, "nm DAQ DOD (final).txt") -> (w213:string)
          n458 = local read "Trace B ?"() -> (w229:bool)
          n459 = Threshold 1D Array(2:w118, 3:w107) -> (0:w117:dbl)  [unwired: 1 in]
          n460 = Threshold 1D Array(2:w119, 3:w107) -> (0:w106:dbl)  [unwired: 1 in]
          n461 = Build Path(base path=w266, name or relative path=w213) -> (appended path=w267:path)
          n462 = Subtract(x=w106, y=w117) -> (x-y=w116:dbl)
          n463 = case shown="True" w229 {
            tunnel: w228 -> [_ _]
            tunnel: [u32 0 ("millisecond timer value") w915] -> w227
            tunnel: w151 -> [_ _]
            frame False {
            }
            frame True {
              w928 = u32 10000  # timeout (10sec)
              # "Note:Closing the serial port allows it to be used by other applications without quitting LabVIEW."
              # "Close session to port."
              # "Configure Serial port (baud rate, data bits, parity, stop bits and flow control)."
              # "Write bytes to port."
              n464 = Wait (ms)(milliseconds to wait=u32 20000) -> (millisecond timer value=w915:u32)
              n465 = local read "Shutter VISA resource name"() -> (w922:refnum<visa-resource-name>)
              n466 = local read "Shutter data bits"() -> (w919:u16)
              n467 = local read "Shutter baud rate"() -> (w921:u32)
              n468 = local read "Shutter parity"() -> (w920:u16)
              n469 = local read "Shutter flow control"() -> (w918:u16)
              n470 = local read "Shutter stop bits"() -> (w917:u16)
              n471 = local read "Shutter open string"() -> (w914:string)
              n472 = call-poly "VISA Configure Serial Port"("VISA resource name"=w922, "timeout (10sec)"=w928, "baud rate (9600)"=w921, "data bits (8)"=w919, "parity (0:none)"=w920, "stop bits (10: 1 bit)"=w917, "flow control (0:none)"=w918) -> ("VISA resource name out"=w927:refnum<visa-resource-name>, "error out"=w926:errorcluster)  [unwired: 2 in, 5 out]
              n473 = VISA Write(VISA resource name=w927, write buffer=w914, error in (no error)=w926) -> (VISA resource name out=w924:refnum<visa-resource-name>, error out=w923:errorcluster)  [unwired: 1 out]
              n474 = VISA Close(VISA resource name=w924, error in (no error)=w923) -> (error out=w925:errorcluster)
              n475 = call <vilib>:"Simple Error Handler.vi"("error in (no error)"=w925) -> ()  [unwired: 1 in, 8 out]
            }
          }
          n476 = Array Subset(array=w109, index=w117, length=w116) -> (w115:dbl[])
          n477 = call-poly <vilib>:"Write To Spreadsheet File.vi"("transpose? (no:F)"=TRUE, "format (%.3f)"="%.9f", "2D data"=w257, "file path (dialog if empty)"=w267) -> ()  [unwired: 4 in, 1 out]
          n478 = call-poly <vilib>:"Mean.vi"("X"=w115) -> ("mean"=w112:dbl)  [unwired: 1 out]
          n479 = case shown="True" w229 {
            tunnel: w237 -> [_ w845]
            tunnel: w227 -> [_ _]
            tunnel: [w795 w805] -> w207
            tunnel: w206 -> [_ w804]
            tunnel: w104 -> [_ w803]
            tunnel: w175 -> [w793 w802]
            tunnel: w174 -> [w792 w801]
            tunnel: [dbl[] [] w797] -> w100
            frame False {
              n480 = call "Close.vi"("error in (no error)"=w792, "VISA resource name"=w793) -> ("error out"=w794:errorcluster)  [unwired: 9 in]
              n481 = call <vilib>:"Simple Error Handler.vi"("error in (no error)"=w794) -> ()  [unwired: 4 in, 5 out]
              n482 = Wait (ms)(milliseconds to wait=u32 1) -> (millisecond timer value=w795:u32)
            }
            frame True {
              # "Scope time axis"
              # "Current wavelength"
              n483 = local read "Final number of\nscope points"() -> (w818:dbl)
              n484 = Initialize Array(0.0 ("element"), w818) -> (w819:dbl[])
              n485 = while {
                tunnel: w802 -> [w855]
                tunnel: [w864] -> w852
                tunnel: w801 -> [w854]
                tunnel: [w863] -> w853
                shift-right: [w882] -> w821
                shift-left: w819 -> [w881]
                shift-right: [w865] -> w800
                shift-left: 0 -> [w866]
                stop <- w878 stop-if-true
                n486 = local read "Channel TAS (0: Channel 1)"() -> (w860:u16)
                n487 = local read "Scope Timeout (ms)"() -> (w861:u32)
                n488 = call "RG Read (Single Waveform) change OPC for WAIT.vi"("error in (no error)"=w854, "Maximum Time (10000ms)"=w861, "Channel (0: Channel 1)"=w860, "VISA resource name"=w855) -> ("error out"=w857:errorcluster, "Waveform Graph"=w859:waveform(dbl), "VISA resource name out"=w858:refnum<visa-resource-name>)  [unwired: 5 in]
                "B trace (Channel1)" <- w859
                n489 = local read "Scope average\nnumber of points"() -> (w883:dbl)
                n490 = Unbundle By Name(w859) -> ("Y"=w876:dbl[])
                n491 = local read "Final number of\nscope points"() -> (w875:dbl)
                n492 = local read "Averages on scope"() -> (w856:i32)
                n493 = call-poly <vilib>:"Decimate (single shot).vi"("averaging"=TRUE, "decimating factor"=w883, "X"=w876) -> ("Decimated Array"=w872:dbl[])  [unwired: 7 in, 1 out]
                n494 = Array Size(array=w872) -> (size(s)=w871:i32)
                n495 = Initialize Array(0.0 ("element"), w875) -> (w873:dbl[])
                n496 = Equal To 0?(x=w871) -> (x = 0?=w868:bool)
                n497 = Select(t=0.0, s=w868, f=w856) -> (s? t:f=w867:dbl)
                n498 = Add(x=w866, y=w867) -> (x+y=w865:dbl)
                "Btrace Readout Counter" <- w865
                n499 = local read "Number of Averages"() -> (w880:i32)
                n500 = Select(t=w873, s=w868, f=w872) -> (s? t:f=w870:dbl[])
                n501 = VISA Write(VISA resource name=w858, write buffer="*WAI", error in (no error)=w857) -> (VISA resource name out=w864:refnum<visa-resource-name>, error out=w863:errorcluster)  [unwired: 1 out]
                n502 = Add(x=w881, y=w870) -> (x+y=w882:dbl[])
                n503 = Greater Or Equal?(x=w865, y=w880) -> (x >= y?=w879:bool)
                n504 = Or(x=w879, y="Stop Btrace Measurement") -> (x .or. y?=w878:bool)
              }
              n505 = Number To Decimal String(number=w804, width (-)=i16 3) -> (decimal integer string=w807:string)
              n506 = Concatenate Strings(w807, "nm Scope CH1 B trace (raw data).txt") -> (w811:string)
              n507 = global read "global tas.vi" "Root Path"() -> (w823:path)
              n508 = Build Path(base path=w823, name or relative path=w811) -> (appended path=w822:path)
              n509 = local read "Averages on scope"() -> (w799:i32)
              n510 = Divide(x=w800, y=w799) -> (x/y=w798:dbl)
              n511 = local read "Scope pretrigger points"() -> (w829:dbl)
              n512 = Divide(x=w821, y=w798) -> (x/y=w820:dbl[])
              n513 = call "Close.vi"("error in (no error)"=w853, "VISA resource name"=w852) -> ("error out"=w851:errorcluster)  [unwired: 9 in]
              n514 = Build Array(w803, w820) -> (w826:dbl[][])
              n515 = call <vilib>:"Simple Error Handler.vi"("error in (no error)"=w851) -> ()  [unwired: 4 in, 5 out]
              n516 = call-poly <vilib>:"Write To Spreadsheet File.vi"("transpose? (no:F)"=TRUE, "format (%.3f)"="%.9f", "2D data"=w826, "file path (dialog if empty)"=w822) -> ()  [unwired: 4 in, 1 out]
              n517 = Multiply(x=w829, y=0.75) -> (x*y=w830:dbl)
              n518 = Array Subset(array=w820, index=0, length=w830) -> (w848:dbl[])
              n519 = Add Array Elements(numeric array=w848) -> (sum=w849:dbl)
              n520 = Divide(x=w849, y=w830) -> (x/y=w850:dbl)
              n521 = local read "Background level (on Amp)"() -> (w815:dbl)
              n522 = Subtract(x=w820, y=w850) -> (x-y=w846:dbl[])
              n523 = local read "Calculate Output Method"() -> (w827:T1)
              n524 = Subtract(x=w845, y=w846) -> (x-y=w816:dbl[])
              n525 = Add(x=w816, y=w815) -> (x+y=w817:dbl[])
              n526 = case shown="\"Kubelka-Munk\"" w827 {
                tunnel: w817 -> [w886 w892 w911]
                tunnel: [w885 w889 w904] -> w797
                frame "Transmission" {
                  # "Calculate output as: deltaOD = log(T/T')"
                  n527 = local read "Background level (on Amp)"() -> (w887:dbl)
                  n528 = Divide(x=w887, y=w886) -> (x/y=w888:dbl[])
                  n529 = Logarithm Base 10(1:w888) -> (0:w885:dbl[])
                }
                frame "Reflectance" {
                  # "Calculate output as: Transient abs. = 1 - RT = (Rbkg - R(t)) / Rbkg"
                  n530 = local read "Background level (on Amp)"() -> (w891:dbl)
                  n531 = Subtract(x=w891, y=w892) -> (x-y=w890:dbl[])
                  n532 = Divide(x=w890, y=w891) -> (x/y=w889:dbl[])
                }
                frame "Kubelka-Munk" {
                  # "Calculate output from\nKM = (1-Rrelative)^2/(2*Rrelative)"
                  n533 = local read "100% Reflectance Standard (V)"() -> (w894:dbl)
                  n534 = local read "Amplification Factor"() -> (w895:dbl)
                  n535 = local read "Background level (on Amp)"() -> (w912:dbl)
                  n536 = Multiply(x=w894, y=w895) -> (x*y=w893:dbl)
                  n537 = Divide(x=w911, y=w893) -> (x/y=w897:dbl[])
                  n538 = Subtract(x=1.0, y=w897) -> (x-y=w899:dbl[])
                  n539 = Divide(x=w912, y=w893) -> (x/y=w906:dbl)
                  n540 = Square(x=w899) -> (x^2=w900:dbl[])
                  n541 = Subtract(x=1.0, y=w906) -> (x-y=w909:dbl)
                  n542 = Multiply(x=w897, y=2.0) -> (x*y=w901:dbl[])
                  n543 = Square(x=w909) -> (x^2=w908:dbl)
                  n544 = Divide(x=w900, y=w901) -> (x/y=w896:dbl[])
                  n545 = Multiply(x=w906, y=2.0) -> (x*y=w907:dbl)
                  n546 = Divide(x=w908, y=w907) -> (x/y=w903:dbl)
                  n547 = Subtract(x=w896, y=w903) -> (x-y=w904:dbl[])
                }
              }
              n548 = local read "Scope Timebase (per div)"() -> (w832:dbl)
              n549 = local read "Scope pretrigger points"() -> (w831:dbl)
              n550 = Divide(x=w832, y=10.0) -> (x/y=w838:dbl)
              n551 = Divide(x=w832, y=w831) -> (x/y=w833:dbl)
              n552 = Multiply(x=w838, y=-1.0) -> (x*y=w835:dbl)
              n553 = To Time Stamp(1:w835) -> (0:w834:timestamp)
              n554 = global read "global tas.vi" "Root Path"() -> (w840:path)
              n555 = Bundle By Name("Y"=w797, "t0"=w834, "dt"=w833) -> (→"Scope CH1 DOD data (A-B final)":waveform(dbl))  [unwired: 1 in]
              n556 = Concatenate Strings(w807, "nm Scope CH1 (final A-B).txt") -> (w809:string)
              n557 = Build Path(base path=w840, name or relative path=w809) -> (appended path=w841:path)
              n558 = Wait (ms)(milliseconds to wait=u32 1) -> (millisecond timer value=w805:u32)
              n559 = Build Array(w803, w797) -> (w839:dbl[][])
              n560 = call-poly <vilib>:"Write To Spreadsheet File.vi"("transpose? (no:F)"=TRUE, "format (%.3f)"="%.9f", "2D data"=w839, "file path (dialog if empty)"=w841) -> ()  [unwired: 4 in, 1 out]
            }
          }
          n561 = Array Subset(array=w100, index=w122) -> (w121:dbl[])  [unwired: 1 in]
          n562 = call-poly <vilib>:"Mean.vi"("X"=w121) -> ("mean"=w113:dbl)  [unwired: 1 out]
          n563 = Subtract(x=w113, y=w112) -> (x-y=w114:dbl)
          n564 = Subtract(x=w100, y=w114) -> (x-y=w111:dbl[])
          n565 = Array Subset(array=w109, index=w106) -> (w110:dbl[])  [unwired: 1 in]
          n566 = Build Array (concatenate)(w111, w110) -> (w108:dbl[])
          n567 = Array Subset(array=w107, index=w106) -> (w105:dbl[])  [unwired: 1 in]
          n568 = Build Array (concatenate)(w104, w105) -> (w103:dbl[])
          n569 = Build Array(w103, w108) -> (w102:dbl[][])
          n570 = global read "global tas.vi" "Root Path"() -> (w129:path)
          n571 = Concatenate Strings(w128, "nm Stitched Scope-DAQ (final A-B).txt") -> (w130:string)
          n572 = Build Path(base path=w129, name or relative path=w130) -> (appended path=w126:path)
          n573 = call-poly <vilib>:"Write Delimited Spreadsheet.vi"("file path (dialog if empty)"=w126, "format (%.3f)"="%.9f", "2D data"=w102, "transpose? (no:F)"=TRUE ("transpose? (F)")) -> ()  [unwired: 10 in, 2 out]
        }
        n574 = flat-sequence {
          tunnel: w61 -> [_]
          frame #0 {
            w94 = FALSE
            n575 = local write "2b - Spectrum"(w94) -> ()
            n576 = local write "2a - Kinetic"(w94) -> ()
            n577 = One Button Dialog(message="Acquisition complete.") -> ()  [unwired: 1 in, 1 out]
          }
        }
      }
      frame 3 {
        # "Code"
        n578 = case shown="False" w1011 {
          tunnel: w1011 -> [w1088 w1102]
          tunnel: [w1085 w1102] -> w1010
          frame False {
            # "PTI Mono"
            n579 = flat-sequence {
              tunnel: [w1095] -> w1089
              tunnel: w1088 -> [w1095]
              tunnel: w1089 -> [w1101]
              tunnel: [w1101] -> w1086
              tunnel: [w1097] -> w1087
              frame #0 {
                # "Check where mono is"
                n580 = call "UserInputMonoValue.vi"() -> ("Monochromator readout"=w1096:dbl)  [unwired: 17 in, 2 out]
                n581 = local write "Current Wavelength (PTI)"(w1096) -> ()
              }
              frame #1 {
                # "Find out which grating is currently being used"
                n582 = Two Button Dialog(message="Please press the appropriate\nbutton for the grating currently\nselected on the monochromator.", 1:"Visible" ("F button name (\"Cancel\")"), 2:"IR" ("T button name (\"OK\")")) -> (T button?=w1097:bool)
                n583 = local write "Is IR"(w1097) -> ()
              }
            }
            n584 = case shown="True" w1087 {
              tunnel: w1086 -> [w1090 w1091]
              tunnel: [w1090 w1091] -> w1085
              frame False {
              }
              frame True {
                n585 = local read "Current Wavelength (PTI)"() -> (w1094:dbl)
                n586 = Multiply(x=w1094, y=2.0) -> (x*y=w1093:dbl)
                n587 = local write "Current Wavelength (PTI)"(w1093) -> ()
              }
            }
          }
          frame True {
            # "Oriel Mono"
          }
        }
        n588 = case shown="True" w1010 {
          tunnel: [w1013 w1073] -> w1012
          frame False {
            # "PTI Mono"
            n589 = flat-sequence {
              tunnel: [w1017] -> w1014
              tunnel: [w1067] -> _
              tunnel: w1014 -> [w1067]
              tunnel: [w1066] -> w1013
              frame #0 {
                n590 = local read "Is IR"() -> (w1016:bool)
                n591 = call "RG Get User Input Wavelength.vi"() -> ("Go to wavelength"=w1015:i32)  [unwired: 11 in]
                n592 = case shown="True" w1016 {
                  tunnel: [w1020 w1043] -> w1017
                  tunnel: w1015 -> [w1019 w1042]
                  tunnel: w1015 -> [w1018 w1041]
                  frame True {
                    # "Currently in IR"
                    n593 = Greater?(x=w1018, y=1000.0) -> (0:w1021:bool)
                    n594 = case shown="True" w1021 {
                      tunnel: [w1024 w1033] -> w1020
                      tunnel: w1019 -> [w1023 w1032]
                      frame False {
                        n595 = stacked-sequence {
                          seq-local: [_ w1029 _] -> [_ _ w1031]
                          tunnel: [_ _ w1031] -> w1024
                          tunnel: w1023 -> [_ w1029 _]
                          frame #0 {
                            # "switch to visible\nand recal mono"
                            n596 = One Button Dialog(message="Please switch\nto the visible grating\nnow.") -> (true=w1025:bool)  [unwired: 1 in]
                            n597 = case shown="True" w1025 {
                              frame False {
                              }
                              frame True {
                                n598 = call "UserInputMonoValue.vi"() -> ("Monochromator readout"=w1027:dbl)  [unwired: 17 in, 2 out]
                                n599 = local write "Is IR"(FALSE ("Is IR")) -> ()
                                n600 = local write "Current Wavelength (PTI)"(w1027) -> ()
                              }
                            }
                          }
                          frame #1 {
                            # "now in visible, move \nto new wavelength"
                            n601 = local read "Current Wavelength (PTI)"() -> (w1030:dbl)
                            n602 = call "ChazMoveMono.vi"("Move to"=w1029, "Current"=w1030) -> ()  [unwired: 8 in, 2 out]
                          }
                          frame #2 {
                            n603 = local write "Current Wavelength (PTI)"(w1031) -> ()
                          }
                        }
                      }
                      frame True {
                        # "Still in IR"
                        n604 = stacked-sequence {
                          seq-local: [w1034 _] -> [_ w1040]
                          tunnel: [_ w1040] -> w1033
                          tunnel: w1032 -> [w1034 _]
                          frame #0 {
                            n605 = local read "Current Wavelength (PTI)"() -> (w1039:dbl)
                            n606 = Divide(x=w1034, y=2.0) -> (x/y=w1035:dbl)
                            n607 = Divide(x=w1039, y=2.0) -> (x/y=w1036:dbl)
                            n608 = call "ChazMoveMono.vi"("Move to"=w1035, "Current"=w1036) -> ()  [unwired: 8 in, 2 out]
                          }
                          frame #1 {
                            n609 = local write "Current Wavelength (PTI)"(w1040) -> ()
                          }
                        }
                      }
                    }
                  }
                  frame False {
                    # "Currently in Visible"
                    n610 = Greater?(x=w1041, y=1000.0) -> (0:w1044:bool)
                    n611 = case shown="True" w1044 {
                      tunnel: [w1047 w1052] -> w1043
                      tunnel: w1042 -> [w1046 w1051]
                      frame False {
                        # "Still in Visible"
                        n612 = stacked-sequence {
                          seq-local: [w1048 _] -> [_ w1050]
                          tunnel: [_ w1050] -> w1047
                          tunnel: w1046 -> [w1048 _]
                          frame #0 {
                            n613 = local read "Current Wavelength (PTI)"() -> (w1049:dbl)
                            n614 = call "ChazMoveMono.vi"("Move to"=w1048, "Current"=w1049) -> ()  [unwired: 8 in, 2 out]
                          }
                          frame #1 {
                            n615 = local write "Current Wavelength (PTI)"(w1050) -> ()
                          }
                        }
                      }
                      frame True {
                        n616 = stacked-sequence {
                          seq-local: [_ w1059 _] -> [_ _ w1065]
                          tunnel: [_ _ w1065] -> w1052
                          tunnel: w1051 -> [_ w1059 _]
                          frame #0 {
                            # "switch to IR\nand recal mono"
                            n617 = One Button Dialog(message="Please switch\nto the IR grating\nnow.") -> (true=w1053:bool)  [unwired: 1 in]
                            n618 = case shown="True" w1053 {
                              frame False {
                              }
                              frame True {
                                n619 = call "UserInputMonoValue.vi"() -> ("Monochromator readout"=w1057:dbl)  [unwired: 17 in, 2 out]
                                n620 = local write "Is IR"(TRUE ("Is IR")) -> ()
                                n621 = Multiply(x=w1057, y=2.0) -> (x*y=w1055:dbl)
                                n622 = local write "Current Wavelength (PTI)"(w1055) -> ()
                              }
                            }
                          }
                          frame #1 {
                            # "now in IR, move \nto new wavelength"
                            n623 = local read "Current Wavelength (PTI)"() -> (w1062:dbl)
                            n624 = Divide(x=w1059, y=2.0) -> (x/y=w1060:dbl)
                            n625 = Divide(x=w1062, y=2.0) -> (x/y=w1061:dbl)
                            n626 = call "ChazMoveMono.vi"("Move to"=w1060, "Current"=w1061) -> ()  [unwired: 8 in, 2 out]
                          }
                          frame #2 {
                            n627 = local write "Current Wavelength (PTI)"(w1065) -> ()
                          }
                        }
                      }
                    }
                  }
                }
              }
              frame #1 {
                n628 = call <vilib>:"General Error Handler.vi"() -> ("error out"=w1066:errorcluster)  [unwired: 11 in, 4 out]
              }
            }
          }
          frame True {
            # "Oriel Mono"
            n629 = call "m_open.vi"() -> ("error out"=w1083:errorcluster, "configuration file path copy"=w1084:path)  [unwired: 2 in]
            n630 = call "GetWave.vi"("error in (no error)"=w1083) -> ("error out"=w1076:errorcluster, "Present Wavelength"=w1072:dbl)  [unwired: 1 in]
            n631 = call "RG Get User Input Wavelength.vi"("Current wavelength"=w1072) -> ("Go to wavelength"=w1071:i32)  [unwired: 10 in]
            n632 = call "getgrat.vi"("error in (no error)"=w1076) -> ("error out"=w1077:errorcluster, "Grating"=→"Grating":i32)  [unwired: 1 in]
            n633 = Less Or Equal?(x=w1071, y=590.0) -> (x <= y?=w1074:bool)
            n634 = Select(t=1.0, s=w1074, f=2.0) -> (s? t:f=w1078:dbl)
            n635 = call "setgrat.vi"("error in (no error)"=w1077, "Grating"=w1078) -> ("error out"=w1075:errorcluster)  [unwired: 1 in]
            n636 = call "gowave.vi"("error in (no error)"=w1075, "Destination Wavelength"=w1071) -> ("error out"=w1070:errorcluster)
            n637 = call "GetWave.vi"("error in (no error)"=w1070) -> ("error out"=w1069:errorcluster, "Present Wavelength"=w1068:dbl)  [unwired: 1 in]
            n638 = local write "Current wavelength (Oriel)"(w1068) -> ()
            n639 = call "m_close.vi"("error in (no error)"=w1069, "configuration file path"=w1084) -> ("error out"=w1073:errorcluster)  [unwired: 1 out]
          }
        }
        n640 = flat-sequence {
          tunnel: w1012 -> [_]
          frame #0 {
            n641 = local write "3 - Move mono"(FALSE ("3 - Move shutter")) -> ()
            n642 = One Button Dialog(message="Wavelength change complete.") -> ()  [unwired: 1 in, 1 out]
          }
        }
      }
    }
  }
